vi "ME_acquire_21_HallSensor.vi"() -> ()   [LabVIEW 2015]
doc: "Use this template to build a producer/consumer design pattern. Use this template when you need to execute a process, such as data analysis, when a data source, such as a triggered acquisition, produces data at an uneven rate and you need to execute the process when the data becomes available."
uses:
  Mode.ctl
  oxford_driver/Oxford Drivers/BUSGEN.LLB/OxfordAddress.ctl
  <vilib>/Analysis/baseanly.llb/Mean (DBL).vi
  <vilib>/DAQmx/read.llb/DAQmx Read (Analog 1D DBL 1Chan NSamp).vi
  <vilib>/DAQmx/create/channels.llb/DAQmx Create Channel (AI-Voltage-Basic).vi
  <vilib>/DAQmx/configure/timing.llb/DAQmx Timing (Sample Clock).vi
  <vilib>/Utility/file.llb/Write Delimited Spreadsheet (DBL).vi
  <vilib>/DAQmx/miscellaneous.llb/DAQmx Fill In Error Info.vi
  <vilib>/express/express arith-compare/Formula/XNode/ExpressFormulaBlockNode.xnode
  <vilib>/Analysis/NI_AALBase.lvlib
panel:
  out "B lag":cluster{dbl[], dbl[]}(graph)
  out "T array":dbl[](array[numeric])
  out "Averaged I(T)":dbl[][](array[numeric])
  in  "Averaged P(T)":dbl[][](array[numeric])
  out "remaining elements 2":T1(array[cluster])
  out "Actual mean":dbl format="%0.6f"
  in  "Averaged dt":dbl[][](array[numeric])
  in  "Averaged P(B)":dbl[][](array[numeric])
  out "LockInR":dbl
  out "deltaUaux":dbl
  out "Hall Resistance (Ohm)":dbl caption="Actual AuxV" step=0.1
  in  "Stop":bool
  out "SaveSweep":bool=TRUE
  out "Measurement File_dn":path
  out "Measurement File_up":path
  out "Measurement File_average":path
  out "Actual Polarization":dbl
  in  "Reset IB?":bool
  in  "First?":bool
  in  "Save Period":dbl=1.0
  out "Averaged I(B)":dbl[][](array[numeric])
  out "P(uC/mm^2)":dbl[](array[numeric])
  in  "Sweep":bool
  out "Offset array":dbl[](array[numeric])
  in  "stop 2":bool
  in  "dB":dbl=0.005
  out "Actual B Field (T)":dbl
  out "Actual Temperature (K)":dbl
  out "Actual Current (pA)":dbl
  in  "Tab Control":T2(tab)
  in  "dt (K)":dbl=0.1
  in  "Max temperature (K)":dbl=20.0
  in  "Min Temperature (K)":dbl=4.5
  out "P(T)":cluster{"yi":dbl[], dbl[]}(graph)
  out "I(T)":cluster{dbl[], dbl[]}(graph)
  in  "Set temperature (K)":dbl=4.5
  in  "Temp Ramping Rate (K/min)":dbl=10.0
  in  "Heater Range":enum16{"Off", "Low", "Medium", "High"}(ring)
  in  "Heater On/Off":bool
  out "Setpoint Temperature (K)":dbl
  out "I(T) /Averaged/":cluster{"B array":dbl[], dbl[]}[](graph)
  out "P(T) /Averaged/":cluster{"B array":dbl[], dbl[]}[](graph)
  out "Up/Down 2":bool
  out "I(B) 3":cluster{dbl[], dbl[]}[](graph)
  out "I(B) /Averaged/":cluster{"B array":dbl[], dbl[]}[](graph)
  out "P(B) /Averaged/":cluster{"B array":dbl[], dbl[]}[](graph)
  out "P(B)":cluster{"yi":dbl[], dbl[]}(graph)
  in  "Set Field (T)":dbl
  in  "Go to Set":bool
  in  "Sweep Rate (T/min)":dbl=2.0 format="%.6f"
  in  "Field To Zero":bool
  out "Target Field":dbl
  in  "Min Field (T)":dbl
  in  "Max Field (T)":dbl=0.15
  in  "Threshold B (T)":dbl
  out "Up/Down":bool
  in  "Magnetic Field array (T)":dbl[](array[numeric])=[0.025, 0.05, 0.075, 0.1, 0.125, 0.15, 0.175, 0.2, 0.225, 0.25, 0.275, 0.3]
  in  "T Sweep Rate Array":dbl[](array[numeric])=[10.0, 20.0]
  in  "Max count array":i32[](array[numeric])=[2, 1, 0, 0, 0, 9, 10, 11, 12]
  in  "secs to wait":dbl=180.0
  out "Wait (s)":dbl
  in  "Directory":string
  out "Finished":bool=TRUE
  out "Step Rate":bool
  out "New":bool=TRUE
  in  "Temperature Array":dbl[](array[numeric])=[4.5, 5.0, 6.0, 7.0, 8.0, 9.0, 10.0, 11.0, 12.0]
  in  "Sweep Rate Array":dbl[](array[numeric])=[2.0, 1.0, 0.5, 0.1, 0.05, 9.0, 10.0, 11.0, 12.0]
  in  "Record ALL":bool
  in  "Max Countl":i32
  out "i":i32
  out "j":i32
  out "Step Temp":bool
  in  "FileName":string
  in  "Measure Noise":bool
  in  "Cycles":i32
  in  "maximum value":dbl=10.0 format="%0.2f"
  in  "minimum value":dbl=-10.0 format="%0.2f"
  in  "physical channels":tag="Dev1/ai1"
  out "PSD (pA/Hz^1/2) Peaks Removed":cluster{"f0":dbl, "df":dbl, "magnitude":dbl[]}(graph)
  out "PSD (pA/Hz^1/2)":cluster{"f0":dbl, "df":dbl, "magnitude":dbl[]}(graph)
  out "Current (pA) Filtered":waveform(dbl)(graph)
  out "Current (pA)":dbl[](graph)
  in  "Samples per channel":i32=1000
  in  "Rate":dbl=1000.0 format="%0.2f"
  in  "Cut-Off Frequency":dbl=100.0 caption="Lower Cut-Off"
  in  "Filter On":bool
  in  "Keithley (IV conv) averaging":i32=10
  in  "Lock_in_Amplifier":refnum<visa-resource-name>="GPIB0::5::INSTR"
  out "Dc offset":dbl
  in  "Calibrate":bool
  in  "IV converter":refnum<visa-resource-name>="GPIB0::20::INSTR"
  in  "Magnetic Field":refnum<visa-resource-name>="GPIB0::19::INSTR"
  out "Time Lag":dbl=0.0500025749206543
  in  "Lake Shore":refnum<visa-resource-name>="GPIB0::11::INSTR"
  in  "Temp Refresh (s)":dbl=0.1
  in  "Sampling rate (Hz)":dbl=10.0
  in  "Gain (V/A)":dbl=1000000000.0
  in  "Sample area (mm^2)":dbl=1.0
  out "Calibration Curve":cluster{dbl[], "Best Linear Fit":dbl[]}[](graph)=[{[0.0, 0.005, 0.01, 0.015, 0.02, 0.025, 0.03, 0.035, 0.04, 0.045, 0.05, 0.055, 0.06, 0.065, 0.07, 0.075, 0.08, 0.085, 0.09, 0.095, 0.1, 0.105, 0.11, 0.115, 0.12, 0.125, 0.13, 0.135, 0.14, 0.145, 0.15, 0.155, 0.16, 0.165, 0.17, 0.175, 0.18, 0.185, 0.19, 0.195, 0.2, 0.205, 0.21, 0.215, 0.22, 0.225, 0.23, 0.235, 0.24, 0.245, 0.25, 0.255, 0.26, 0.265, 0.27, 0.275, 0.28, 0.285, 0.29, 0.295, 0.3, 0.305, 0.31, 0.315, 0.32, 0.325, 0.33, 0.335, 0.34, 0.345, 0.35, 0.355, 0.36, 0.365, 0.37, 0.375, 0.38, 0.385, 0.39, 0.395, 0.4, 0.405, 0.41, 0.415, 0.42, 0.425, 0.43, 0.435, 0.44, 0.445, 0.45, 0.455, 0.46, 0.465, 0.47, 0.475, 0.48, 0.485, 0.49, 0.495, 0.5], "Best Linear Fit"=[-1.7e-06, 1.18e-05, 3.66e-05, 6.17e-05, 9.39e-05, 0.000122, 0.0001511, 0.0001781, 0.0002061, 0.0002355, 0.0002616, 0.0002895, 0.0003184, 0.0003446, 0.0003689, 0.0003958, 0.0004207, 0.0004464, 0.0004684, 0.0004953, 0.0005218, 0.0005459, 0.0005692, 0.0005897, 0.0006131, 0.0006347, 0.0006589, 0.0006834, 0.0007035, 0.0007249, 0.0007465, 0.000765, 0.0007858, 0.0008103, 0.0008302, 0.0008467, 0.000868, 0.0008855, 0.0009079, 0.0009248, 0.0009452, 0.0009633, 0.0009828, 0.0009992, 0.0010189, 0.0010338, 0.001054, 0.0010692, 0.0010858, 0.0011036, 0.0011162, 0.0011356, 0.0011502, 0.0011643, 0.0011834, 0.0011985, 0.0012131, 0.0012277, 0.0012423, 0.0012571, 0.0012691, 0.0012827, 0.0012976, 0.001313, 0.0013264, 0.0013388, 0.0013518, 0.0013638, 0.0013782, 0.0013909, 0.0014035, 0.0014175, 0.0014295, 0.0014407, 0.0014538, 0.0014641, 0.0014752, 0.0014861, 0.0014978, 0.0015081, 0.0015203, 0.001532, 0.0015422, 0.0015526, 0.001563, 0.0015754, 0.0015844, 0.0015955, 0.0016056, 0.001614, 0.0016239, 0.0016342, 0.0016457, 0.0016542, 0.0016635, 0.001674, 0.001681, 0.0016886, 0.0016986, 0.0017063, 0.0017155]}, {[0.0, 0.005, 0.01, 0.015, 0.02, 0.025, 0.03, 0.035, 0.04, 0.045, 0.05, 0.055, 0.06, 0.065, 0.07, 0.075, 0.08, 0.085, 0.09, 0.095, 0.1, 0.105, 0.11, 0.115, 0.12, 0.125, 0.13, 0.135, 0.14, 0.145, 0.15, 0.155, 0.16, 0.165, 0.17, 0.175, 0.18, 0.185, 0.19, 0.195, 0.2, 0.205, 0.21, 0.215, 0.22, 0.225, 0.23, 0.235, 0.24, 0.245, 0.25, 0.255, 0.26, 0.265, 0.27, 0.275, 0.28, 0.285, 0.29, 0.295, 0.3, 0.305, 0.31, 0.315, 0.32, 0.325, 0.33, 0.335, 0.34, 0.345, 0.35, 0.355, 0.36, 0.365, 0.37, 0.375, 0.38, 0.385, 0.39, 0.395, 0.4, 0.405, 0.41, 0.415, 0.42, 0.425, 0.43, 0.435, 0.44, 0.445, 0.45, 0.455, 0.46, 0.465, 0.47, 0.475, 0.48, 0.485, 0.49, 0.495, 0.5], "Best Linear Fit"=[-1.7e-06, 1.18e-05, 3.66e-05, 6.17e-05, 9.39e-05, 0.000122, 0.0001511, 0.0001781, 0.0002061, 0.0002355, 0.0002616, 0.0002895, 0.0003184, 0.0003446, 0.0003689, 0.0003958, 0.0004207, 0.0004464, 0.0004684, 0.0004953, 0.0005218, 0.0005459, 0.0005692, 0.0005897, 0.0006131, 0.0006347, 0.0006589, 0.0006834, 0.0007035, 0.0007249, 0.0007465, 0.000765, 0.0007858, 0.0008103, 0.0008302, 0.0008467, 0.000868, 0.0008855, 0.0009079, 0.0009248, 0.0009452, 0.0009633, 0.0009828, 0.0009992, 0.0010189, 0.0010338, 0.001054, 0.0010692, 0.0010858, 0.0011036, 0.0011162, 0.0011356, 0.0011502, 0.0011643, 0.0011834, 0.0011985, 0.0012131, 0.0012277, 0.0012423, 0.0012571, 0.0012691, 0.0012827, 0.0012976, 0.001313, 0.0013264, 0.0013388, 0.0013518, 0.0013638, 0.0013782, 0.0013909, 0.0014035, 0.0014175, 0.0014295, 0.0014407, 0.0014538, 0.0014641, 0.0014752, 0.0014861, 0.0014978, 0.0015081, 0.0015203, 0.001532, 0.0015422, 0.0015526, 0.001563, 0.0015754, 0.0015844, 0.0015955, 0.0016056, 0.001614, 0.0016239, 0.0016342, 0.0016457, 0.0016542, 0.0016635, 0.001674, 0.001681, 0.0016886, 0.0016986, 0.0017063, 0.0017155]}]
  in  "Offset?":bool
  in  "Magnet":bool=TRUE
  in  "Ramp":bool=TRUE
  in  "DaQ":bool
  in  "Moving average":i8=10
  in  "Sample Rate":dbl=1000.0
  in  "Number of Samples":i32=100
  in  "Physical Channel":tag="kartya/ai0"
  in  "Min Voltage":dbl=-5.0
  in  "Max Voltage":dbl=5.0
  in  "Terminal Configuration":i32(ring)=-1 items=["default"=-1, "RSE"=10083, "NRSE"=10078, "Differential"=10106, "Pseudodifferential"=12529]
  out "Confirm":bool
  in  "Dwell Time (ms)":u32=1000
  out "Calibration Curve Data":dbl[][](array[numeric])=[[0.0, 0.005, 0.01, 0.015, 0.02, 0.025, 0.03, 0.035, 0.04, 0.045, 0.05, 0.055, 0.06, 0.065, 0.07, 0.075, 0.08, 0.085, 0.09, 0.095, 0.1, 0.105, 0.11, 0.115, 0.12, 0.125, 0.13, 0.135, 0.14, 0.145, 0.15, 0.155, 0.16, 0.165, 0.17, 0.175, 0.18, 0.185, 0.19, 0.195, 0.2, 0.205, 0.21, 0.215, 0.22, 0.225, 0.23, 0.235, 0.24, 0.245, 0.25, 0.255, 0.26, 0.265, 0.27, 0.275, 0.28, 0.285, 0.29, 0.295, 0.3, 0.305, 0.31, 0.315, 0.32, 0.325, 0.33, 0.335, 0.34, 0.345, 0.35, 0.355, 0.36, 0.365, 0.37, 0.375, 0.38, 0.385, 0.39, 0.395, 0.4, 0.405, 0.41, 0.415, 0.42, 0.425, 0.43, 0.435, 0.44, 0.445, 0.45, 0.455, 0.46, 0.465, 0.47, 0.475, 0.48, 0.485, 0.49, 0.495, 0.5], [-1.7e-06, 1.18e-05, 3.66e-05, 6.17e-05, 9.39e-05, 0.000122, 0.0001511, 0.0001781, 0.0002061, 0.0002355, 0.0002616, 0.0002895, 0.0003184, 0.0003446, 0.0003689, 0.0003958, 0.0004207, 0.0004464, 0.0004684, 0.0004953, 0.0005218, 0.0005459, 0.0005692, 0.0005897, 0.0006131, 0.0006347, 0.0006589, 0.0006834, 0.0007035, 0.0007249, 0.0007465, 0.000765, 0.0007858, 0.0008103, 0.0008302, 0.0008467, 0.000868, 0.0008855, 0.0009079, 0.0009248, 0.0009452, 0.0009633, 0.0009828, 0.0009992, 0.0010189, 0.0010338, 0.001054, 0.0010692, 0.0010858, 0.0011036, 0.0011162, 0.0011356, 0.0011502, 0.0011643, 0.0011834, 0.0011985, 0.0012131, 0.0012277, 0.0012423, 0.0012571, 0.0012691, 0.0012827, 0.0012976, 0.001313, 0.0013264, 0.0013388, 0.0013518, 0.0013638, 0.0013782, 0.0013909, 0.0014035, 0.0014175, 0.0014295, 0.0014407, 0.0014538, 0.0014641, 0.0014752, 0.0014861, 0.0014978, 0.0015081, 0.0015203, 0.001532, 0.0015422, 0.0015526, 0.001563, 0.0015754, 0.0015844, 0.0015955, 0.0016056, 0.001614, 0.0016239, 0.0016342, 0.0016457, 0.0016542, 0.0016635, 0.001674, 0.001681, 0.0016886, 0.0016986, 0.0017063, 0.0017155]]
  in  "Temp/Magnetic Field":bool
  out "index":i8
  out "Read?":bool
  out "Magnetic Field (T)":dbl[](array[numeric])
  out "Reset":bool
  out "Measured Current (pA)":dbl[](array[numeric])
  out "Elapsed Time (s)":dbl[](array[numeric])
  out "Start time":timestamp
  in  "Enum":T3=enum."Process"
  out "B array":dbl[](array[numeric])
  in  "dB (T)":dbl=0.0025
  in  "Counter":i8
  out "L magnet (H)":dbl
  out "R magnet (mOhm)":dbl
  out "Actual Current (R0)":dbl
  out "Nominal Field (T)":dbl
  out "Temperature array":dbl[](array[numeric])
  in  "New Measurement File":bool
  out "Measurement File":path
  out "refnum out":refnum<file>
  in  "Measuring":bool
  in  "Measure /Pause":bool
  in  "stop":bool
  # "DeltaForce"
  # "Discrete"
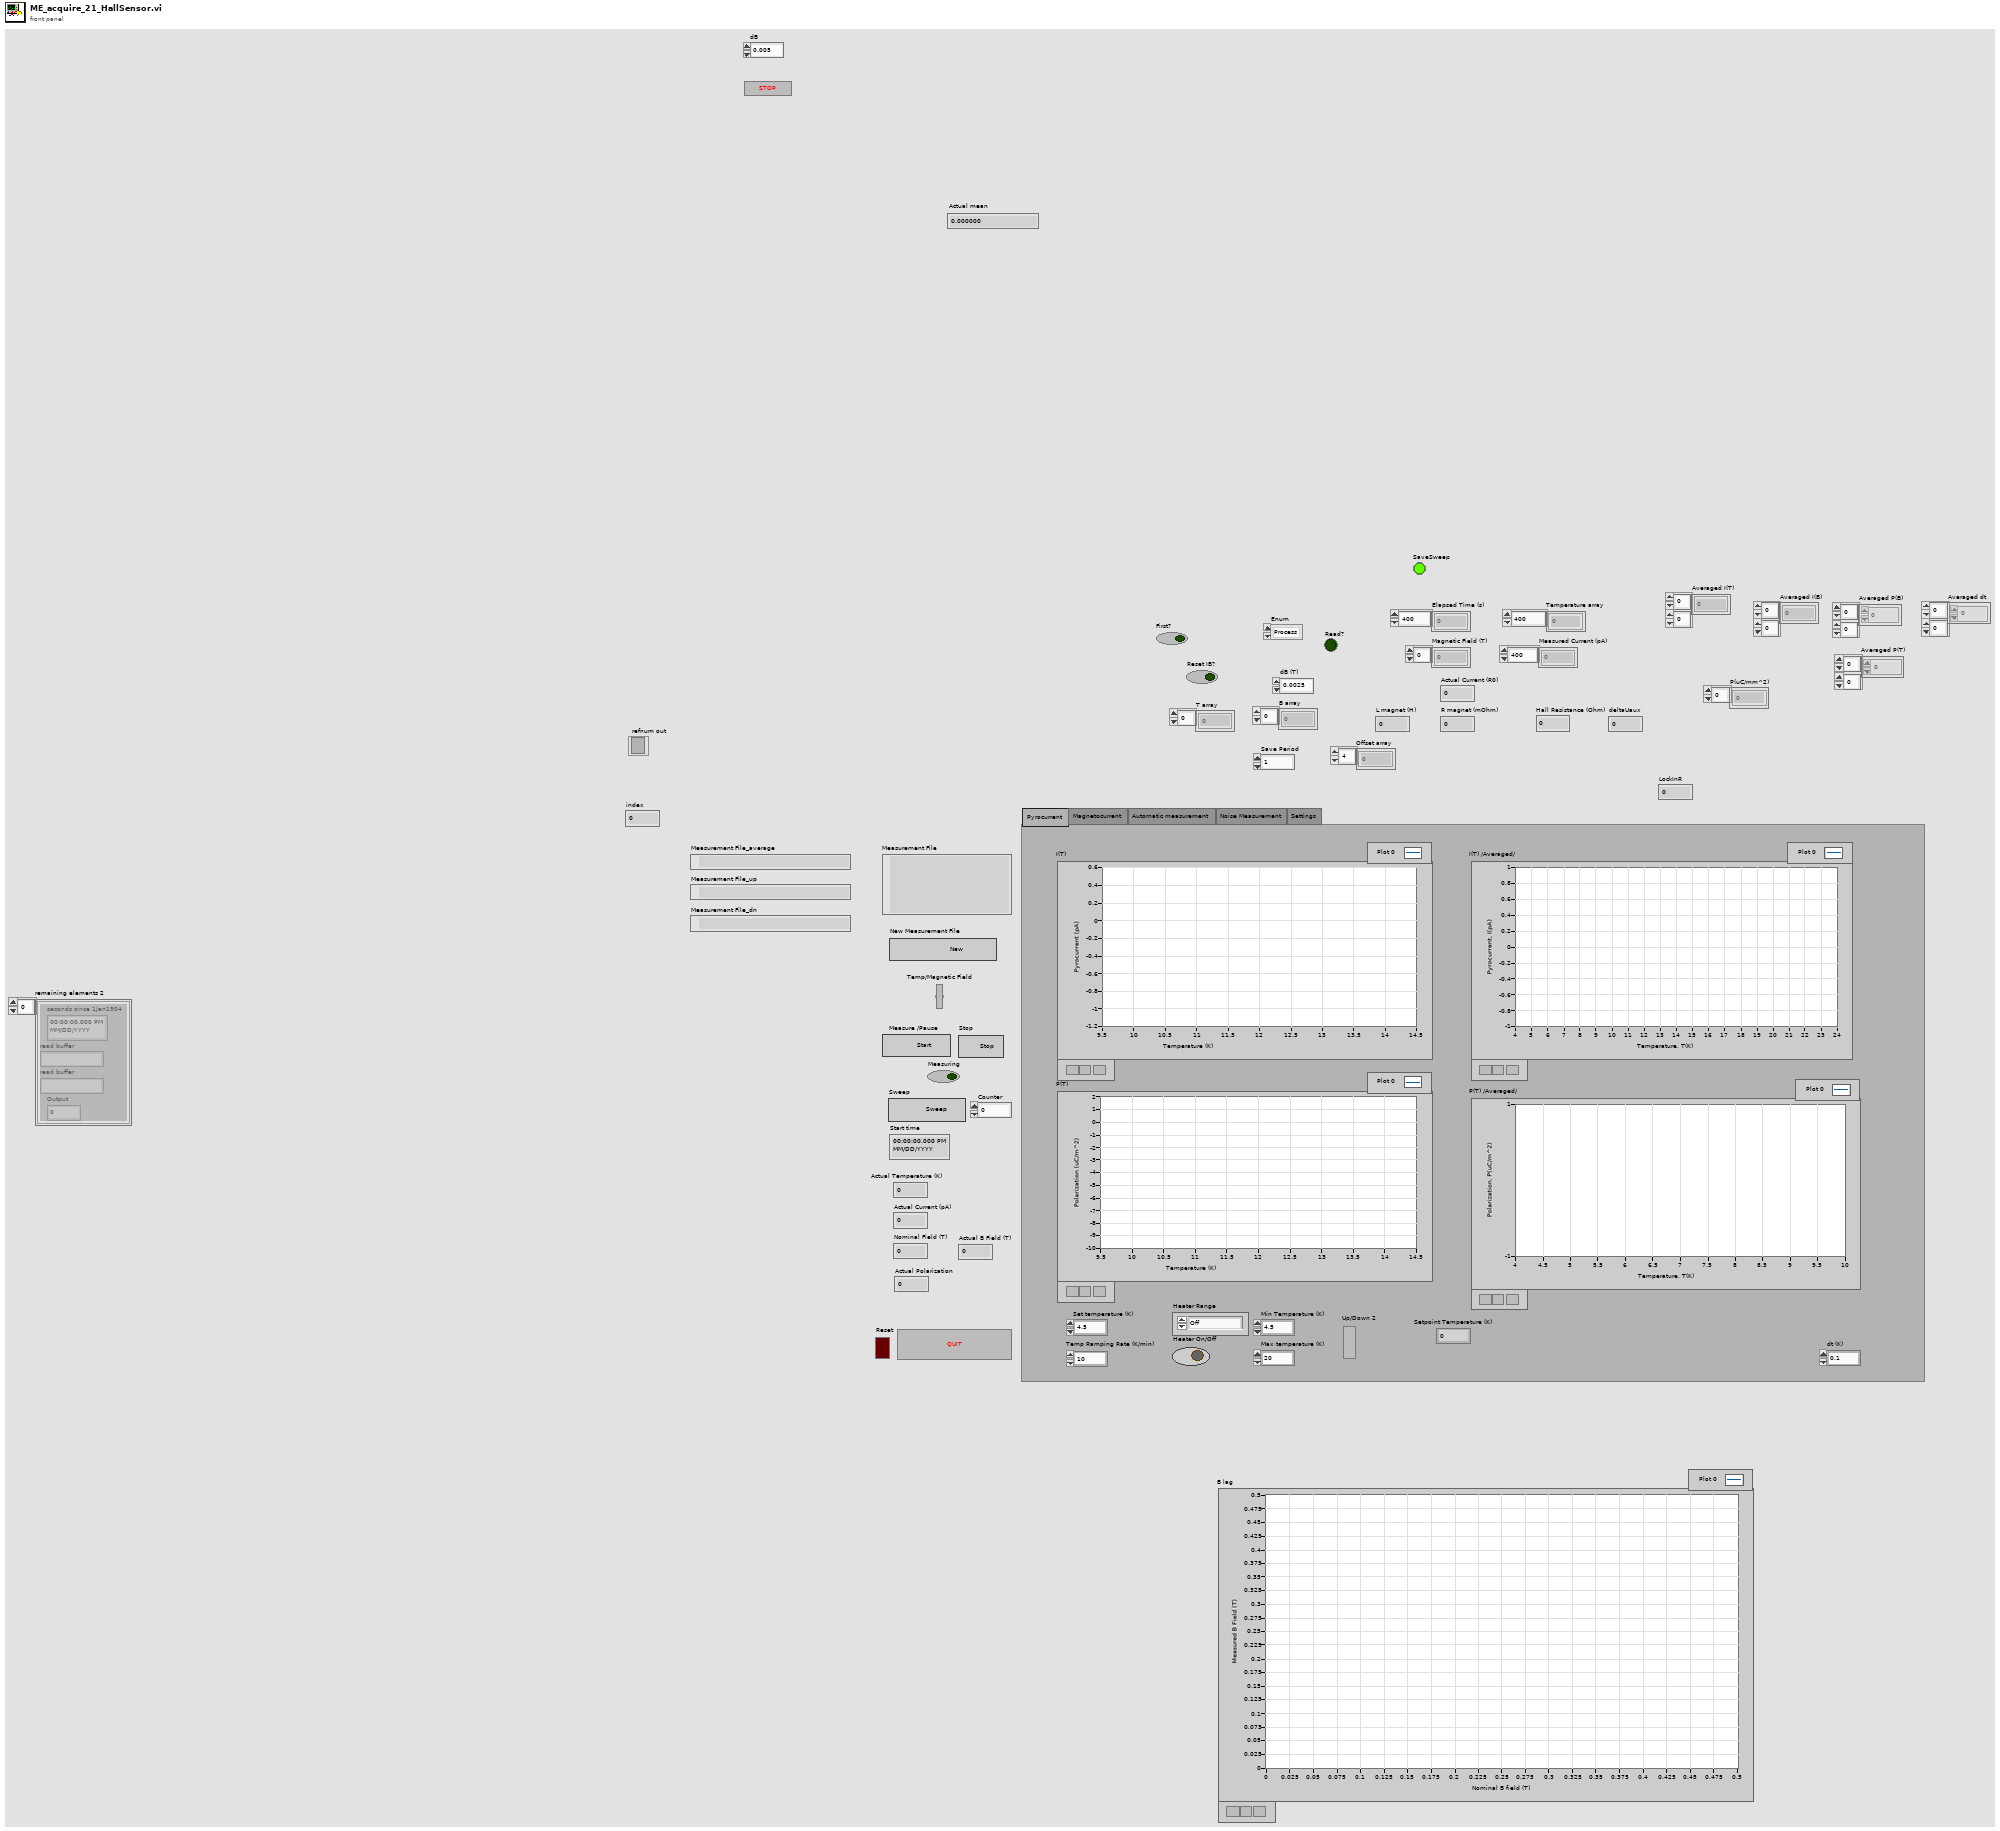
[diagram p1: front panel]
types:
  T1 = cluster{"seconds since 1Jan1904":timestamp, "read buffer":string, "read buffer":string, "Output":dbl}[]
  T2 = enum32{"Pyrocurrent", "Magnetocurrent", "Automatic measurement", "Noise Measurement", "Settings"}
  T3 = typedef "Mode.ctl" = enum16{"Offset", "Process", "Sweep", "StepOxford", "StepDelta", "Plot", "Save", "New", "Return", ""}
  T4 = cluster{"seconds since 1Jan1904":timestamp, "read buffer":string, "read buffer":string, "Output":dbl}
  T5 = enum16{"open", "replace", "create", "open or create", "replace or create", "replace or create with confirmation"}
  T6 = typedef "OxfordAddress.ctl" = cluster{"Com Port":i32, "ISOBUS Address":i32, "GPIB Address":i16, "Communication":enum16{"RS232", "ISOBUS", "GPIB", "Gateway"}}
  T7 = cluster{"B array":dbl[], "Averaged P(B) Out":dbl[]}
  T8 = cluster{"B array":dbl[], "BaselineSubtracted I(B)":dbl[]}
  T9 = cluster{"B array":dbl[], "Averaged P(B) Out":dbl[]}[]
  T10 = cluster{"B array":dbl[], "BaselineSubtracted I(B)":dbl[]}[]
  T11 = cluster{"T array":dbl[], "Averaged P(T) Out":dbl[]}
  T12 = cluster{"T array":dbl[], "Averaged I(B) out":dbl[]}
  T13 = cluster{"T array":dbl[], "Averaged P(T) Out":dbl[]}[]
  T14 = cluster{"T array":dbl[], "Averaged I(B) out":dbl[]}[]
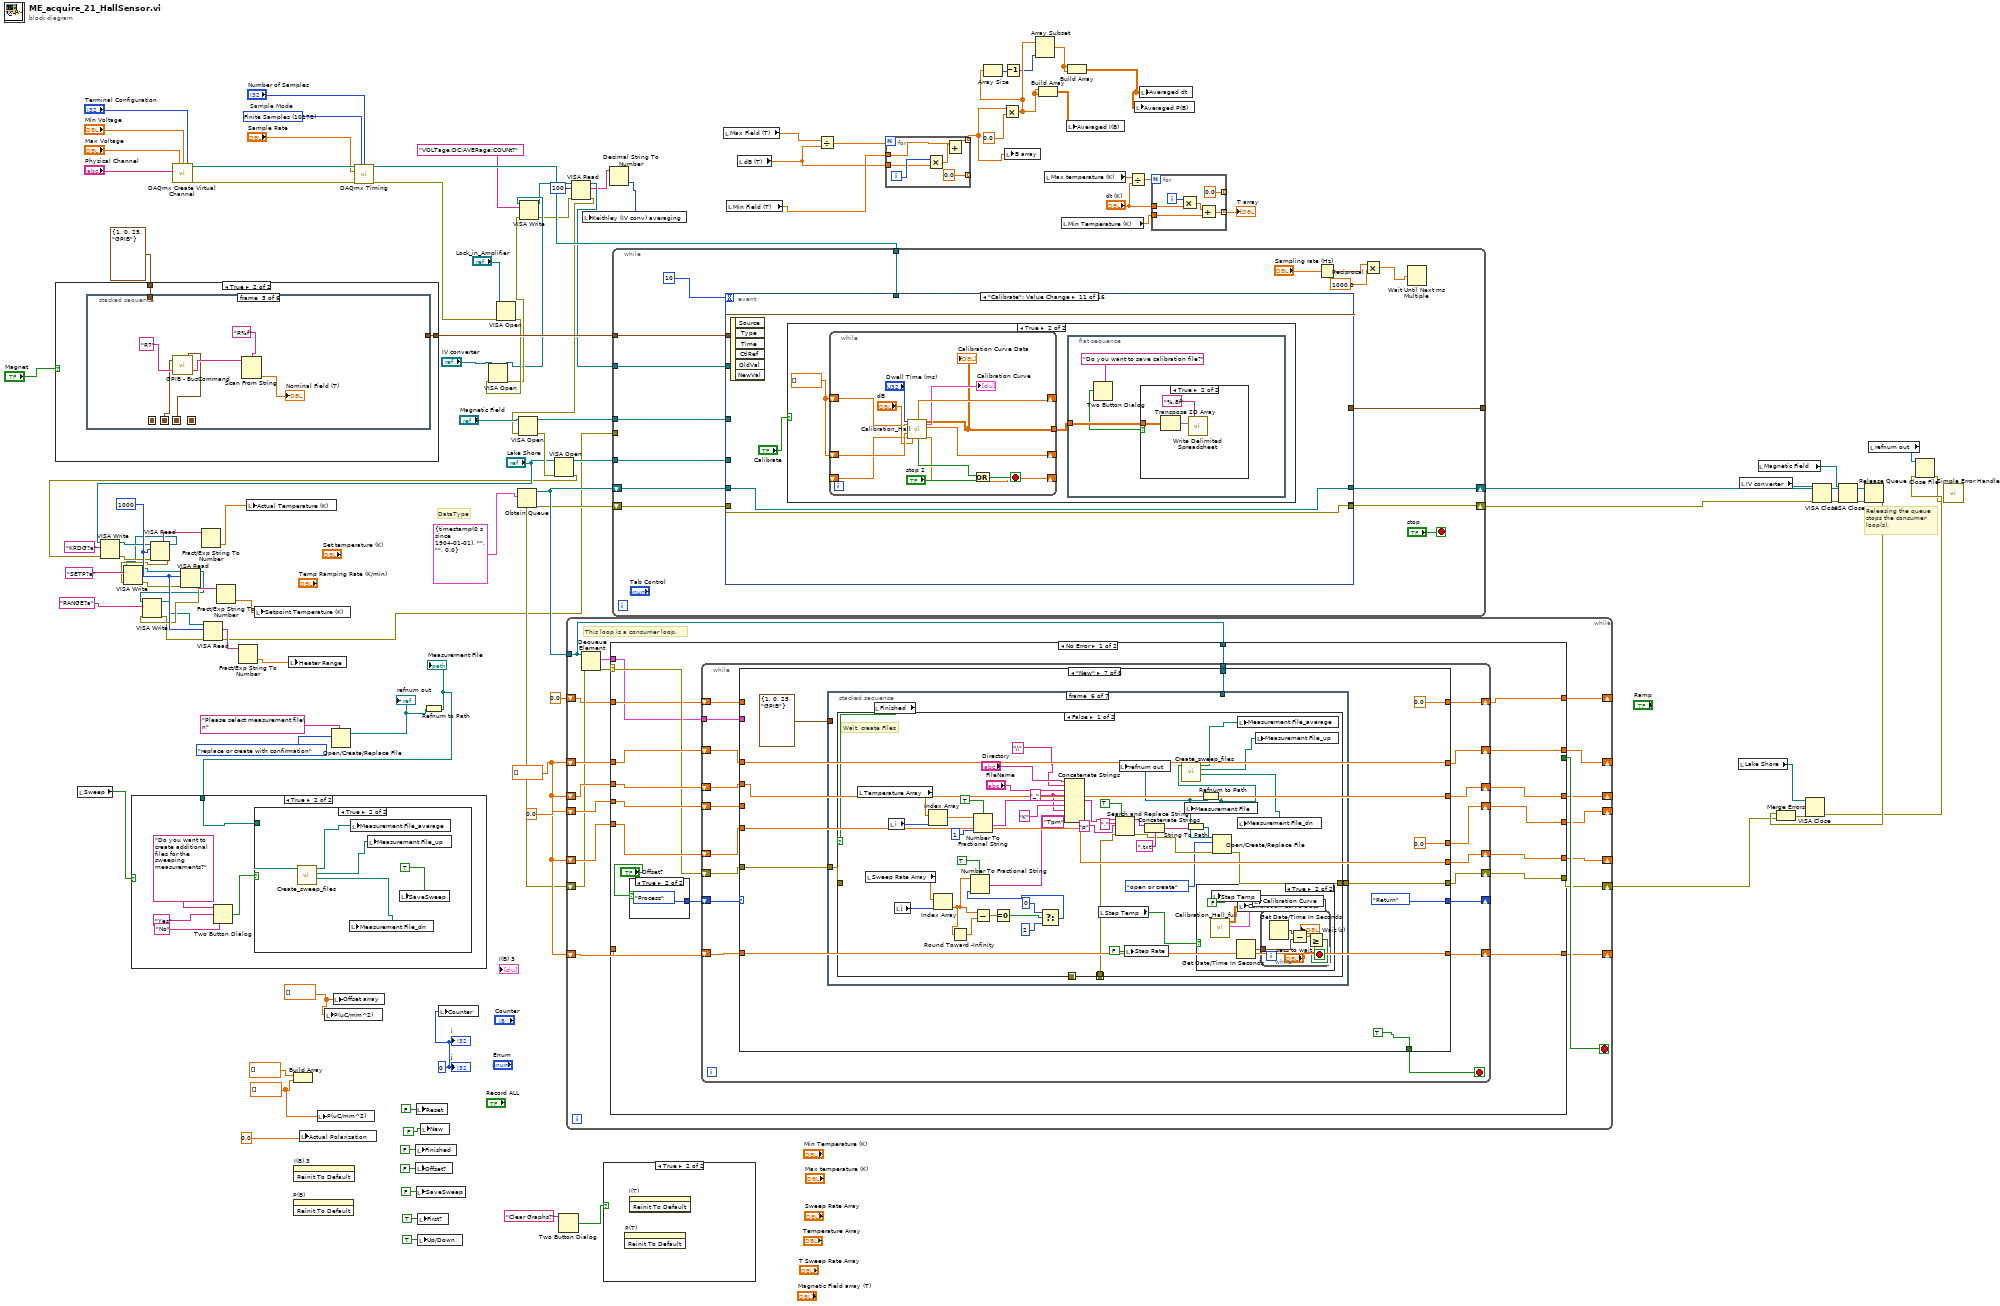
[diagram p0: block diagram]
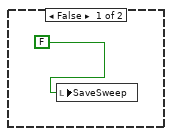
[diagram p4: hidden frame]
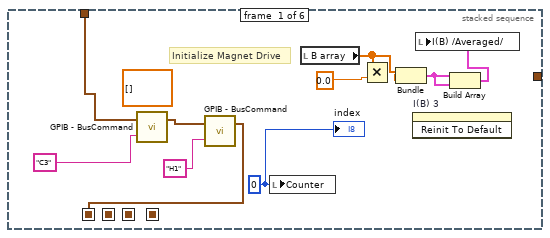
[diagram p6: hidden frame]
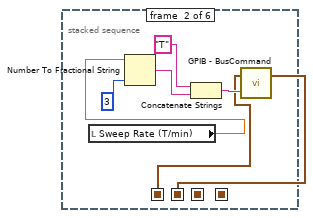
[diagram p7: hidden frame]
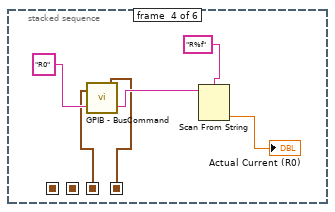
[diagram p8: hidden frame]
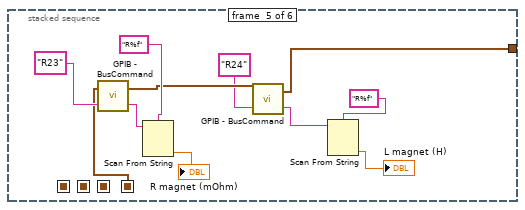
[diagram p9: hidden frame]
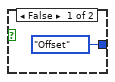
[diagram p11: hidden frame]
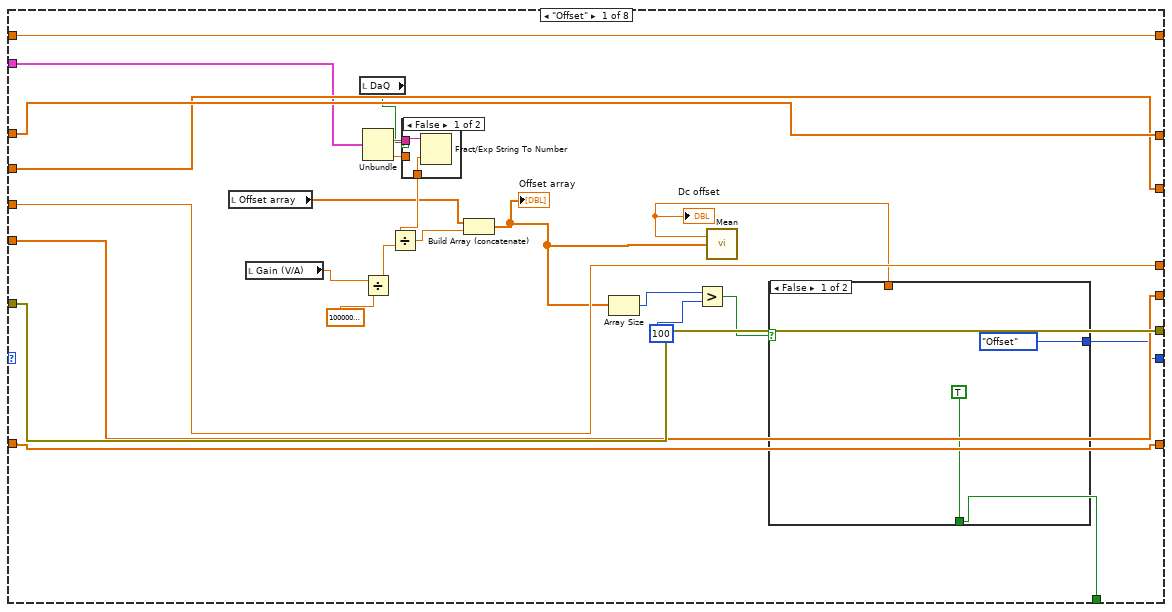
[diagram p12: hidden frame]
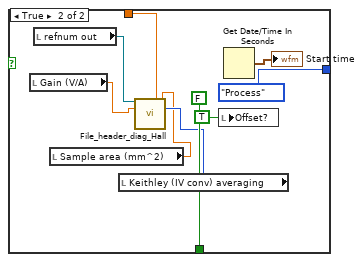
[diagram p14: hidden frame]
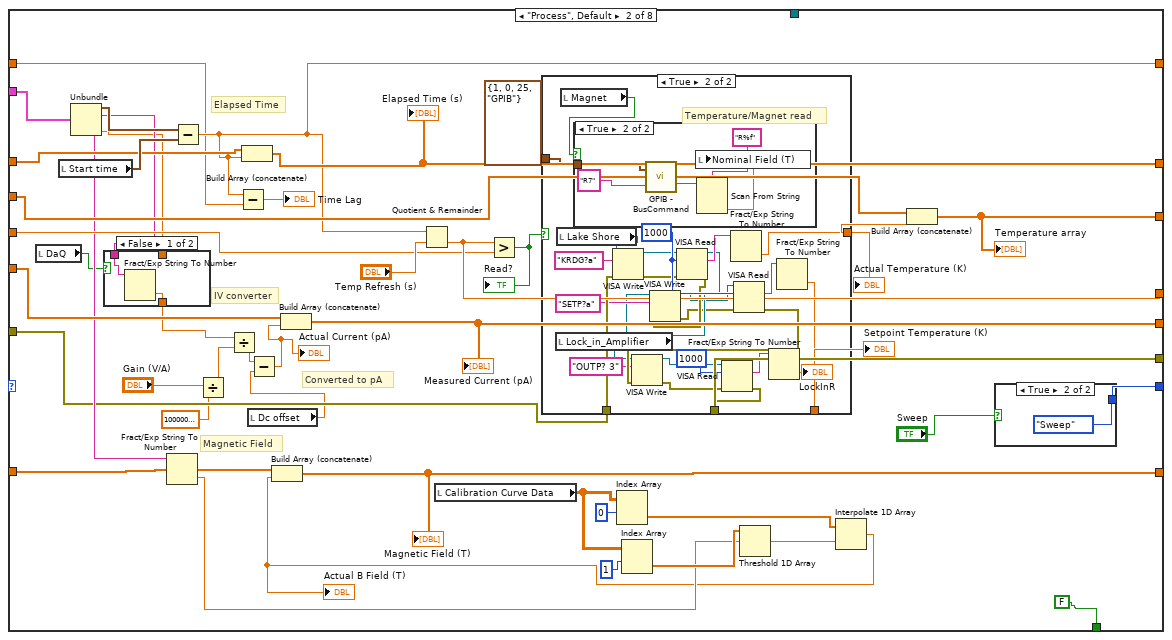
[diagram p15: hidden frame]
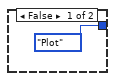
[diagram p17: hidden frame]
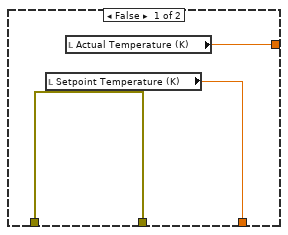
[diagram p18: hidden frame]
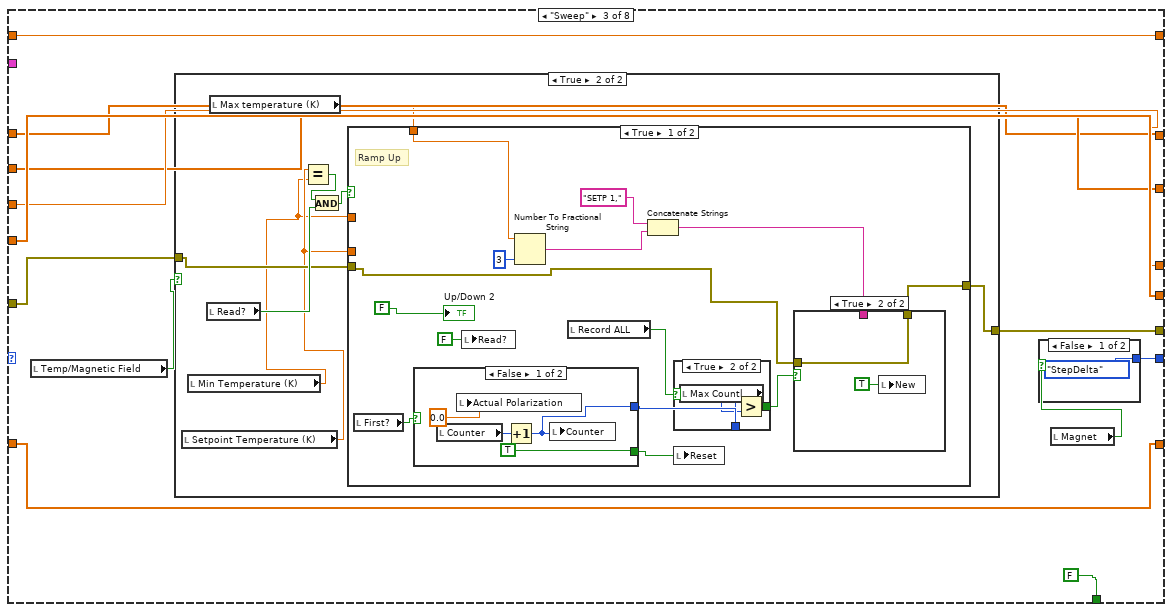
[diagram p20: hidden frame]
diagram:
  w27 = 10178 items=["Finite Samples"=10178, "Continuous Samples"=10123, "Hardware Timed Single Point"=12522]  # Sample Mode
  w54 = u32 1000 ("byte count")
  w65 = 0 ("j")
  w62 = dbl[] []
  w80 = dbl[] []
  w86 = dbl[] []
  # "DataType"
  # "Releasing the queue stops the consumer loop(s)."
  n1 = case shown="True" "Magnet" {
    tunnel: T6 {"Com Port"=1, "ISOBUS Address"=0, "GPIB Address"=25, "Communication"=enum."GPIB"} ("Address") -> [w110 w112]
    tunnel: [w110 w111] -> w92
    frame False {
    }
    frame True {
      n2 = stacked-sequence {
        seq-local: [w120 _ _ _ _ _] -> [_ w125 _ _ _ _]
        seq-local: [_ w124 _ _ _ _] -> [_ _ w132 _ _ _]
        seq-local: [_ _ w131 _ _ _] -> [_ _ _ w138 _ _]
        seq-local: [_ _ _ w137 _ _] -> [_ _ _ _ w149 _]
        tunnel: w112 -> [w122 _ _ _ _ _]
        tunnel: [_ _ _ _ w147 _] -> w111
        frame #0 {
          (unwired) dbl[][] []
          w118 = i8 0 ("Counter")
          # "Initialize Magnet Drive"
          n3 = call "GPIB - BusCommand.vi"("Command"="C3", "Address"=w122) -> ("Address(thru)"=w121:T6)  [unwired: 1 out]
          n4 = call "GPIB - BusCommand.vi"("Command"="H1", "Address"=w121) -> ("Address(thru)"=w120:T6)  [unwired: 1 out]
          n5 = local write "Counter"(w118) -> ()
          n6 = local read "B array"() -> (w116:dbl[])
          n7 = Multiply(x=w116, y=0.0) -> (x*y=w115:dbl[])
          n8 = Bundle("B array"=w116, w115) -> (w114:cluster{"B array":dbl[], dbl[]})  [unwired: 1 in]
          n9 = invoke on="I(B) 3" class="XYGraph (strict)" method="Reinit To Default"() -> ()  [unwired: 3 in, 3 out]
          n10 = Build Array(w114, w114) -> (w113:cluster{"B array":dbl[], dbl[]}[])
          n11 = local write "I(B) /Averaged/"(w113) -> ()
          "index" <- w118
        }
        frame #1 {
          n12 = local read "Sweep Rate (T/min)"() -> (w126:dbl)
          n13 = Number To Fractional String(number=w126, precision (6)=i16 3) -> (F-format string=w128:string)  [unwired: 2 in]
          n14 = Concatenate Strings("T" ("format string"), w128) -> (w127:string)
          n15 = call "GPIB - BusCommand.vi"("Command"=w127, "Address"=w125) -> ("Address(thru)"=w124:T6)  [unwired: 1 out]
        }
        frame #2 {
          n16 = call "GPIB - BusCommand.vi"("Command"="R7" ("format string"), "Address"=w132) -> ("Reply"=w136:string, "Address(thru)"=w131:T6)
          n17 = Scan From String(format string="R%f" ("remaining string"), input string=w136) -> (output 1=→"Nominal Field (T)":dbl)  [unwired: 3 in, 3 out]
        }
        frame #3 {
          n18 = call "GPIB - BusCommand.vi"("Command"="R0" ("format string"), "Address"=w138) -> ("Reply"=w142:string, "Address(thru)"=w137:T6)
          n19 = Scan From String(format string="R%f" ("remaining string"), input string=w142) -> (output 1=→"Actual Current (R0)":dbl)  [unwired: 3 in, 3 out]
        }
        frame #4 {
          n20 = call "GPIB - BusCommand.vi"("Command"="R23" ("format string"), "Address"=w149) -> ("Reply"=w153:string, "Address(thru)"=w148:T6)
          n21 = Scan From String(format string="R%f" ("remaining string"), input string=w153) -> (output 1=→"R magnet (mOhm)":dbl)  [unwired: 3 in, 3 out]
          n22 = call "GPIB - BusCommand.vi"("Command"="R24" ("format string"), "Address"=w148) -> ("Reply"=w145:string, "Address(thru)"=w147:T6)
          n23 = Scan From String(format string="R%f" ("remaining string"), input string=w145) -> (output 1=→"L magnet (H)":dbl)  [unwired: 3 in, 3 out]
        }
        frame #5 {
        }
      }
    }
  }
  n24 = local read "Sweep"() -> (w70:bool)
  n25 = call-poly <vilib>:"DAQmx Create Virtual Channel.vi"("maximum value"="Max Voltage", "minimum value"="Min Voltage", "input terminal configuration"="Terminal Configuration", "physical channels"="Physical Channel") -> ("task out"=w25:refnum<k21>, "error out"=w26:errorcluster)  [unwired: 10 in]
  n26 = Build Array(dbl[] [], w62) -> ()  [unwired: 1 out]
  n27 = invoke on="P(B)" class="XYGraph (strict)" method="Reinit To Default"() -> ()  [unwired: 3 in, 3 out]
  n28 = invoke on="I(B) 3" class="XYGraph (strict)" method="Reinit To Default"() -> ()  [unwired: 3 in, 3 out]
  n29 = local write "Actual Polarization"(0.0 ("Actual Polarization")) -> ()
  n30 = local write "P(uC/mm^2)"(w62) -> ()
  n31 = local write "P(uC/mm^2)"(w80) -> ()
  n32 = Open/Create/Replace File(prompt="Please select measurement file\n", operation (0:open)=T5."replace or create with confirmation") -> (refnum out=w89:refnum<file>)  [unwired: 4 in, 2 out]
  "refnum out" <- w89
  n33 = local write "Offset array"(w80) -> ()
  n34 = call-poly <vilib>:"DAQmx Timing.vi"("task/channels in"=w25, "sample mode"=w27, "samples per channel"="Number of Samples", "rate"="Sample Rate", "error in"=w26) -> ("task out"=w17:refnum<k21>, "error out"=w18:errorcluster)  [unwired: 9 in]
  n35 = local write "Finished"(FALSE ("Finished")) -> ()
  n36 = local write "Offset?"(FALSE ("Offset?")) -> ()
  n37 = local write "Reset"(FALSE ("Reset")) -> ()
  n38 = local write "SaveSweep"(FALSE ("SaveSweep")) -> ()
  n39 = local write "First?"(TRUE ("First?")) -> ()
  n40 = local write "Up/Down"(TRUE ("Up/Down")) -> ()
  n41 = local write "New"(FALSE ("New")) -> ()
  n42 = Refnum to Path(1:w89) -> (0:w69:path)
  "Measurement File" <- w69
  n43 = case shown="True" w70 {
    tunnel: w69 -> [_ w154]
    frame False {
    }
    frame True {
      n44 = Two Button Dialog(message="Do you want to create additional files for the sweeping measurements?" ("string"), 1:"No" ("F button name (\"Cancel\")"), 2:"Yes" ("T button name (\"OK\")")) -> (T button?=w156:bool)
      n45 = case shown="True" w156 {
        tunnel: w154 -> [_ w164]
        frame False {
          n46 = local write "SaveSweep"(FALSE ("SaveSweep")) -> ()
        }
        frame True {
          n47 = call "Create_sweep_files.vi"("Measurement File"=w164) -> ("Path 3"=w161:path, "Path 2"=w162:path, "Path"=w163:path)  [unwired: 8 in]
          n48 = local write "Measurement File_dn"(w161) -> ()
          n49 = local write "Measurement File_average"(w163) -> ()
          n50 = local write "Measurement File_up"(w162) -> ()
          n51 = local write "SaveSweep"(TRUE) -> ()
        }
      }
    }
  }
  n52 = local write "Counter"(w65) -> ()
  n53 = VISA Open(error in (no error)=w18, VISA resource name="Lock_in_Amplifier") -> (error out=w37:errorcluster)  [unwired: 3 in, 1 out]
  n54 = VISA Open(error in (no error)=w37, VISA resource name="IV converter") -> (VISA resource name=w14:refnum<visa-resource-name>, error out=w15:errorcluster)  [unwired: 3 in]
  n55 = Obtain Queue(element data type=T4 {"seconds since 1Jan1904"=timestamp(0 s since 1904-01-01), "read buffer"="", "read buffer"="", "Output"=0.0} ("output cluster")) -> (queue out=w109:refnum<queue>, error out=w84:errorcluster)  [unwired: 4 in, 1 out]
  n56 = VISA Write(VISA resource name=w14, write buffer="VOLTage:DC:AVERage:COUNt?", error in (no error)=w15) -> (VISA resource name out=w10:refnum<visa-resource-name>, error out=w12:errorcluster)  [unwired: 1 out]
  n57 = Two Button Dialog(message="Clear Graphs?") -> (T button?=w64:bool)  [unwired: 2 in]
  n58 = while {
    tunnel: w109 -> [w165]
    shift-right: [w178] -> _
    shift-left: w86 -> [w177]
    shift-right: [w176] -> _
    shift-left: w86 -> [w175]
    shift-right: [w174] -> _
    shift-left: w86 -> [w173]
    shift-right: [w172] -> _
    shift-left: 0.0 -> [w171]
    shift-right: [w170] -> _
    shift-left: w86 -> [w169]
    shift-right: [w179] -> w97
    shift-left: w84 -> [w168]
    shift-right: [w167] -> _
    shift-left: 0.0 -> [w166]
    stop <- w180 stop-if-true
    # "This loop is a consumer loop."
    n59 = Dequeue Element(queue=w165, error in (no error)=w168) -> (element=w181:T4, error out=w182:errorcluster)  [unwired: 1 in, 2 out]
    n60 = case shown="No Error" w182 {
      selector: w182 -> [w189 w898]
      tunnel: w181 -> [w183 _]
      tunnel: [_ TRUE] -> w180
      tunnel: [w188 w898] -> w179
      tunnel: [w199 w897] -> w178
      tunnel: w177 -> [w198 w897]
      tunnel: [w197 w894] -> w176
      tunnel: w175 -> [w196 w894]
      tunnel: [w195 w893] -> w174
      tunnel: w173 -> [w194 w893]
      tunnel: [w193 w895] -> w172
      tunnel: w171 -> [w192 w895]
      tunnel: [w191 w896] -> w170
      tunnel: w169 -> [w190 w896]
      tunnel: [w187 w892] -> w167
      tunnel: w166 -> [w186 w892]
      tunnel: w165 -> [w184 _]
      frame No Error {
        n61 = case shown="True" "Offset?" {
          tunnel: [Mode."Offset" ("Enum") Mode."Process" ("Enum")] -> w200
          frame False {
          }
          frame True {
          }
        }
        n62 = while {
          shift-right: [w209] -> _
          shift-left: w200 -> [w221]
          tunnel: w183 -> [w220]
          shift-right: [w219] -> w199
          shift-left: w198 -> [w218]
          shift-right: [w211] -> w191
          shift-left: w190 -> [w210]
          shift-right: [w213] -> w193
          shift-left: w192 -> [w212]
          shift-right: [w217] -> w197
          shift-left: w196 -> [w216]
          shift-right: [w207] -> w188
          shift-left: w189 -> [w208]
          shift-right: [w215] -> w195
          shift-left: w194 -> [w214]
          shift-right: [w205] -> w187
          shift-left: w186 -> [w204]
          tunnel: w184 -> [w203]
          stop <- w206 stop-if-true
          n63 = case shown="\"New\"" w221 {
            selector: w221 -> [_ _ _ _ _ _ _ w885]
            tunnel: w220 -> [w239 w302 _ _ _ _ _ _]
            tunnel: [w245 w299 w348 w482 w538 w611 w724 w890] -> w219
            tunnel: w218 -> [w245 w294 w348 w482 w538 w607 w724 w890]
            tunnel: [w240 w298 w351 w479 w540 w613 w722 w887] -> w217
            tunnel: w216 -> [w240 w297 w351 w479 w540 w608 w722 w887]
            tunnel: [w241 w296 w353 w477 w535 w614 w720 w884] -> w215
            tunnel: w214 -> [w241 w295 w353 w477 w535 w609 w720 w884]
            tunnel: [w243 w293 w350 w480 w536 w617 0.0 w888] -> w213
            tunnel: w212 -> [w243 w292 w350 w480 w536 w617 _ w888]
            tunnel: [w244 w289 w349 w481 w537 w612 w723 w889] -> w211
            tunnel: w210 -> [w244 w290 w349 w481 w537 w610 w723 w889]
            tunnel: [w228 w287 w346 Mode."Plot" ("Enum") Mode."Save" ("Enum") w618 Mode."Return" ("Enum") w885] -> w209
            tunnel: w208 -> [w242 w285 w355 w474 w543 w616 w716 w886]
            tunnel: [w242 w284 w354 w473 w543 w616 w715 w886] -> w207
            tunnel: [w224 FALSE FALSE FALSE FALSE w605 TRUE TRUE] -> w206
            tunnel: [w227 w281 w347 w475 w539 w615 0.0 w891] -> w205
            tunnel: w204 -> [w227 w280 w347 w475 w539 w615 _ w891]
            tunnel: w203 -> [_ _ _ _ _ _ w714 _]
            frame "Offset" {
              n64 = local read "Offset array"() -> (w233:dbl[])
              n65 = local read "Gain (V/A)"() -> (w237:dbl)
              n66 = local read "DaQ"() -> (w223:bool)
              n67 = Unbundle(w239) -> ("read buffer"=w226:string, "Output"=w222:dbl)  [unwired: 2 out]
              n68 = Divide(x=w237, y=1000000000000.0) -> (x/y=w235:dbl)
              n69 = case shown="False" w223 {
                tunnel: [w247 w248] -> w238
                tunnel: w226 -> [w246 _]
                tunnel: w222 -> [_ w248]
                frame False {
                  n70 = Fract/Exp String To Number(string=w246) -> (number=w247:dbl)  [unwired: 3 in, 1 out]
                }
                frame True {
                }
              }
              n71 = Divide(x=w238, y=w235) -> (x/y=w234:dbl)
              n72 = Build Array (concatenate)(w233, w234) -> (w229:dbl[])
              "Offset array" <- w229
              n73 = Array Size(array=w229) -> (size(s)=w232:i32)
              n74 = Greater?(x=w232, y=100) -> (0:w230:bool)
              n75 = call-poly <vilib>:"Mean.vi"("X"=w229) -> ("mean"=w225:dbl)  [unwired: 1 out]
              "Dc offset" <- w225
              n76 = case shown="False" w230 {
                tunnel: [Mode."Offset" ("Enum") Mode."Process" ("Enum")] -> w228
                tunnel: w225 -> [_ w255]
                tunnel: [TRUE FALSE] -> w224
                frame False {
                }
                frame True {
                  n77 = local read "Gain (V/A)"() -> (w256:dbl)
                  n78 = local read "refnum out"() -> (w257:refnum<file>)
                  n79 = local read "Sample area (mm^2)"() -> (w251:dbl)
                  n80 = local read "Keithley (IV conv) averaging"() -> (w252:i32)
                  n81 = call "File_header_diag_Hall.vi"("Byte Stream File in"=w257, "OFFSET"=w255, "Sample area"=w251, "Gain"=w256, "Averaging"=w252) -> ()  [unwired: 11 in]
                  n82 = local write "Offset?"(TRUE ("Offset?")) -> ()
                  n83 = Get Date/Time In Seconds() -> (seconds since 1Jan1904=→"Start time":timestamp)
                }
              }
            }
            frame "Process", Default {
              # "Converted to pA"
              # "Magnetic Field"
              # "IV converter"
              # "Elapsed Time"
              n84 = local read "DaQ"() -> (w270:bool)
              n85 = local read "Start time"() -> (w300:timestamp)
              n86 = Unbundle(w302) -> ("seconds since 1Jan1904"=w301:timestamp, "read buffer"=w271:string, "read buffer"=w286:string, "Output"=w268:dbl)
              n87 = case shown="False" w270 {
                tunnel: w271 -> [w306 _]
                tunnel: [w305 w307] -> w269
                tunnel: w268 -> [_ w307]
                frame False {
                  n88 = Fract/Exp String To Number(string=w306) -> (number=w305:dbl)  [unwired: 3 in, 1 out]
                }
                frame True {
                }
              }
              n89 = Fract/Exp String To Number(string=w286) -> (number=w263:dbl)  [unwired: 3 in, 1 out]
              n90 = Subtract(x=w301, y=w300) -> (x-y=w281:dbl)
              n91 = Divide(x="Gain (V/A)", y=1000000000000.0) -> (x/y=w279:dbl)
              n92 = Divide(x=w269, y=w279) -> (x/y=w276:dbl)
              n93 = Subtract(x=w281, y=w280) -> (x-y=→"Time Lag":dbl)
              n94 = Build Array (concatenate)(w294, w281) -> (w299:dbl[])
              "Elapsed Time (s)" <- w299
              n95 = local read "Dc offset"() -> (w274:dbl)
              n96 = Subtract(x=w276, y=w274) -> (x-y=w275:dbl)
              "Actual Current (pA)" <- w275
              n97 = Build Array (concatenate)(w297, w275) -> (w298:dbl[])
              "Measured Current (pA)" <- w298
              n98 = Quotient & Remainder(x=w281, y="Temp Refresh (s)") -> (floor(x/y)=w293:dbl)  [unwired: 1 out]
              n99 = local read "Calibration Curve Data"() -> (w265:dbl[][])
              n100 = Greater?(x=w293, y=w292) -> (0:w291:bool)
              "Read?" <- w291
              n101 = case shown="True" w291 {
                tunnel: [w311 w336] -> w288
                tunnel: w285 -> [w312 w335]
                tunnel: [w312 w315] -> w284
                tunnel: T6 {"Com Port"=1, "ISOBUS Address"=0, "GPIB Address"=25, "Communication"=enum."GPIB"} ("Address") -> [_ w334]
                tunnel: [w310 w330] -> w272
                frame False {
                  n102 = local read "Setpoint Temperature (K)"() -> (w310:dbl)
                  n103 = local read "Actual Temperature (K)"() -> (w311:dbl)
                }
                frame True {
                  w331 = u32 1000 ("byte count")
                  # "Temperature/Magnet read"
                  n104 = local read "Lock_in_Amplifier"() -> (w319:refnum<visa-resource-name>)
                  n105 = local read "Lake Shore"() -> (w333:refnum<visa-resource-name>)
                  n106 = local read "Magnet"() -> (w322:bool)
                  n107 = case shown="True" w322 {
                    tunnel: w334 -> [_ w340]
                    frame False {
                    }
                    frame True {
                      n108 = call "GPIB - BusCommand.vi"("Command"="R7" ("format string"), "Address"=w340) -> ("Reply"=w341:string)  [unwired: 1 out]
                      n109 = Scan From String(format string="R%f" ("remaining string"), input string=w341) -> (output 1=w339:dbl)  [unwired: 3 in, 3 out]
                      n110 = local write "Nominal Field (T)"(w339) -> ()
                    }
                  }
                  n111 = VISA Write(VISA resource name=w333, write buffer="KRDG?a", error in (no error)=w335) -> (VISA resource name out=w329:refnum<visa-resource-name>, error out=w327:errorcluster)  [unwired: 1 out]
                  n112 = VISA Read(VISA resource name=w329, byte count=w331, error in (no error)=w327) -> (VISA resource name out=w328:refnum<visa-resource-name>, read buffer=w337:string, error out=w326:errorcluster)  [unwired: 1 out]
                  n113 = VISA Write(VISA resource name=w328, write buffer="SETP?a", error in (no error)=w326) -> (VISA resource name out=w324:refnum<visa-resource-name>, error out=w325:errorcluster)  [unwired: 1 out]
                  n114 = Fract/Exp String To Number(string=w337) -> (number=w336:dbl)  [unwired: 3 in, 1 out]
                  n115 = VISA Read(VISA resource name=w324, byte count=w331, error in (no error)=w325) -> (read buffer=w323:string, error out=w321:errorcluster)  [unwired: 2 out]
                  n116 = VISA Write(VISA resource name=w319, write buffer="OUTP? 3", error in (no error)=w321) -> (VISA resource name out=w318:refnum<visa-resource-name>, error out=w320:errorcluster)  [unwired: 1 out]
                  n117 = VISA Read(VISA resource name=w318, byte count=u32 1000, error in (no error)=w320) -> (read buffer=w314:string, error out=w315:errorcluster)  [unwired: 2 out]
                  n118 = Fract/Exp String To Number(string=w314) -> (number=→"LockInR":dbl)  [unwired: 3 in, 1 out]
                  n119 = Fract/Exp String To Number(string=w323) -> (number=w330:dbl)  [unwired: 3 in, 1 out]
                }
              }
              "Actual Temperature (K)" <- w288
              "Setpoint Temperature (K)" <- w272
              n120 = Index Array(array=w265, index (row)=0) -> (element=w261:dbl[])  [unwired: 1 in]
              n121 = Index Array(array=w265, index (row)=1 ("index (col)")) -> (element=w264:dbl[])  [unwired: 1 in]
              n122 = Threshold 1D Array(2:w263, 3:w264) -> (0:w262:dbl)  [unwired: 1 in]
              n123 = Interpolate 1D Array(1:w262, 2:w261) -> (0:w260:dbl)
              "Actual B Field (T)" <- w260
              n124 = Build Array (concatenate)(w295, w260) -> (w296:dbl[])
              "Magnetic Field (T)" <- w296
              n125 = Build Array (concatenate)(w290, w288) -> (w289:dbl[])
              "Temperature array" <- w289
              n126 = case shown="True" "Sweep" {
                tunnel: [Mode."Plot" ("Enum") Mode."Sweep" ("Enum")] -> w287
                frame False {
                }
                frame True {
                }
              }
            }
            frame "Sweep" {
              n127 = local read "Temp/Magnetic Field"() -> (w345:bool)
              n128 = case shown="True" w345 {
                tunnel: w355 -> [w364 w421]
                tunnel: [w363 w420] -> w354
                frame False {
                  n129 = local read "Nominal Field (T)"() -> (w359:dbl)
                  n130 = local read "Min Field (T)"() -> (w358:dbl)
                  n131 = local read "Max Field (T)"() -> (w365:dbl)
                  n132 = local read "Read?"() -> (w362:bool)
                  n133 = Greater Or Equal?(x=w358, y=w359) -> (x >= y?=w361:bool)
                  n134 = Compound Arithmetic op=AND(w361, w362) -> (w360:bool)
                  n135 = case shown="False" w360 {
                    tunnel: [w368 w404] -> w363
                    tunnel: w365 -> [w366 w403]
                    tunnel: w358 -> [_ w402]
                    tunnel: w359 -> [_ w400]
                    tunnel: w364 -> [w369 w399]
                    frame True {
                      # "Ramp Up"
                      n136 = case shown="True" "First?" {
                        tunnel: [TRUE ("Save") FALSE ("Save")] -> w372
                        tunnel: [w391 w395] -> w371
                        frame False {
                          n137 = local read "Counter"() -> (w394:i8)
                          n138 = local write "Actual Polarization"(0.0 ("Actual Polarization")) -> ()
                          n139 = Increment(x=w394) -> (x+1=w391:i8)
                          n140 = local write "Counter"(w391) -> ()
                        }
                        frame True {
                          n141 = local read "Counter"() -> (w395:i8)
                          n142 = local write "First?"(FALSE ("First?")) -> ()
                        }
                      }
                      "Reset" <- w372
                      n143 = local write "Read?"(FALSE ("Read?")) -> ()
                      n144 = local read "Record ALL"() -> (w367:bool)
                      n145 = case shown="True" w367 {
                        tunnel: w371 -> [_ w379]
                        tunnel: [FALSE w377] -> w370
                        frame False {
                        }
                        frame True {
                          n146 = Greater?(x=w379, y="Max Countl") -> (0:w377:bool)
                        }
                      }
                      n147 = case shown="True" w370 {
                        tunnel: w369 -> [w383 w390]
                        tunnel: [w382 w390] -> w368
                        tunnel: w366 -> [w381 _]
                        frame False {
                          n148 = local read "Magnet"() -> (w380:bool)
                          n149 = case shown="True" w380 {
                            tunnel: w383 -> [w384 w387]
                            tunnel: [w384 w386] -> w382
                            tunnel: w381 -> [_ w385]
                            frame False {
                            }
                            frame True {
                              n150 = call "Set_B.vi"("error in (no error)"=w387, "address string"="25", "Set Field (T)"=w385) -> ("error out"=w386:errorcluster)  [unwired: 8 in]
                            }
                          }
                          "Target Field" <- w381
                        }
                        frame True {
                          "New" <- TRUE
                        }
                      }
                      "Up/Down" <- FALSE ("Up/Down")
                    }
                    frame False {
                      n151 = Less Or Equal?(x=w403, y=w400) -> (x <= y?=w401:bool)
                      n152 = case shown="True" w401 {
                        tunnel: [w405 w409] -> w404
                        tunnel: w402 -> [_ w407]
                        tunnel: w399 -> [w405 w410]
                        frame False {
                        }
                        frame True {
                          # "Resetting at the end of every cycle"
                          # "Ramp Dn"
                          n153 = local write "Up/Down"(TRUE ("Up/Down")) -> ()
                          n154 = local read "Magnet"() -> (w406:bool)
                          n155 = local write "Target Field"(w407) -> ()
                          n156 = local write "Reset"(TRUE ("Reset")) -> ()
                          n157 = case shown="True" w406 {
                            tunnel: w410 -> [w412 w415]
                            tunnel: [w412 w414] -> w409
                            tunnel: w407 -> [_ w413]
                            frame False {
                            }
                            frame True {
                              n158 = call "Set_B.vi"("error in (no error)"=w415, "address string"="25", "Set Field (T)"=w413) -> ("error out"=w414:errorcluster)  [unwired: 8 in]
                            }
                          }
                        }
                      }
                      n159 = local write "Read?"(FALSE ("Read?")) -> ()
                    }
                  }
                }
                frame True {
                  n160 = local read "Setpoint Temperature (K)"() -> (w419:dbl)
                  n161 = local read "Min Temperature (K)"() -> (w418:dbl)
                  n162 = local read "Read?"() -> (w424:bool)
                  n163 = local read "Max temperature (K)"() -> (w417:dbl)
                  n164 = Equal?(x=w419, y=w418) -> (x = y?=w422:bool)
                  n165 = And(x=w422, y=w424) -> (x .and. y?=w423:bool)
                  n166 = case shown="True" w423 {
                    tunnel: [w425 w462] -> w420
                    tunnel: w417 -> [w433 w461]
                    tunnel: w418 -> [_ w460]
                    tunnel: w419 -> [_ w458]
                    tunnel: w421 -> [w426 w457]
                    frame True {
                      # "Ramp Up"
                      n167 = local read "First?"() -> (w437:bool)
                      n168 = case shown="False" w437 {
                        tunnel: [TRUE ("Save") FALSE ("Save")] -> w428
                        tunnel: [w449 w455] -> w431
                        frame False {
                          n169 = local read "Counter"() -> (w452:i8)
                          n170 = local write "Actual Polarization"(0.0 ("Actual Polarization")) -> ()
                          n171 = Increment(x=w452) -> (x+1=w449:i8)
                          n172 = local write "Counter"(w449) -> ()
                        }
                        frame True {
                          n173 = local read "Counter"() -> (w455:i8)
                          n174 = local write "First?"(FALSE ("First?")) -> ()
                        }
                      }
                      n175 = local write "Read?"(FALSE ("Read?")) -> ()
                      n176 = Number To Fractional String(number=w433, precision (6)=i16 3) -> (F-format string=w435:string)  [unwired: 2 in]
                      n177 = local read "Record ALL"() -> (w432:bool)
                      n178 = Concatenate Strings("SETP 1," ("write buffer"), w435) -> (w427:string)
                      n179 = case shown="True" w432 {
                        tunnel: w431 -> [_ w448]
                        tunnel: [FALSE w447] -> w429
                        frame False {
                        }
                        frame True {
                          n180 = local read "Max Countl"() -> (w446:i32)
                          n181 = Greater?(x=w448, y=w446) -> (0:w447:bool)
                        }
                      }
                      n182 = local write "Reset"(w428) -> ()
                      n183 = case shown="True" w429 {
                        tunnel: w427 -> [w442 _]
                        tunnel: w426 -> [w440 w443]
                        tunnel: [w439 w443] -> w425
                        frame False {
                          n184 = local read "Lake Shore"() -> (w441:refnum<visa-resource-name>)
                          n185 = VISA Write(VISA resource name=w441, write buffer=w442, error in (no error)=w440) -> (error out=w439:errorcluster)  [unwired: 2 out]
                        }
                        frame True {
                          n186 = local write "New"(TRUE ("New")) -> ()
                        }
                      }
                      "Up/Down 2" <- FALSE ("Up/Down")
                    }
                    frame False {
                      n187 = Equal?(x=w461, y=w458) -> (x = y?=w459:bool)
                      n188 = case shown="True" w459 {
                        tunnel: [w463 w467] -> w462
                        tunnel: w460 -> [_ w466]
                        tunnel: w457 -> [w463 w468]
                        frame False {
                        }
                        frame True {
                          w464 = TRUE ("Reset")
                          # "Ramp Dn"
                          n189 = local write "Up/Down 2"(w464) -> ()
                          n190 = Number To Fractional String(number=w466, precision (6)=i16 3) -> (F-format string=w470:string)  [unwired: 2 in]
                          n191 = local write "Reset"(w464) -> ()
                          n192 = local read "Lake Shore"() -> (w465:refnum<visa-resource-name>)
                          n193 = Concatenate Strings("SETP 1," ("write buffer"), w470) -> (w472:string)
                          n194 = VISA Write(VISA resource name=w465, write buffer=w472, error in (no error)=w468) -> (error out=w467:errorcluster)  [unwired: 2 out]
                        }
                      }
                      n195 = local write "Read?"(FALSE ("Read?")) -> ()
                    }
                  }
                }
              }
              n196 = local read "Magnet"() -> (w344:bool)
              n197 = case shown="False" w344 {
                tunnel: [Mode."StepDelta" ("Enum") Mode."Plot" ("Enum")] -> w346
                frame False {
                }
                frame True {
                }
              }
            }
            frame "StepDelta" {
              n198 = flat-sequence {
                tunnel: w474 -> [w489]
                tunnel: [w488] -> w473
                frame #0 {
                  # "Check if it is time to step Field"
                  n199 = local read "Sweep Rate (T/min)"() -> (w490:dbl)
                  n200 = local read "Time Lag"() -> (w486:dbl)
                  n201 = xnode "Sweep Delay"("SweepRate"=w490, "Resolution"=0.001 ("Voltage Step (V)")) -> ("Result"=w487:dbl)  [unwired: 2 in, 1 out]
                  n202 = Divide(x=w486, y=w487) -> (x/y=w484:dbl)
                  n203 = Multiply(x=0.001 ("y"), y=w484) -> (x*y=w483:dbl)
                  "deltaUaux" <- w483
                  n204 = stacked-sequence {
                    tunnel: w489 -> [_ w501]
                    tunnel: [_ w500] -> w488
                    tunnel: w483 -> [w495 _]
                    frame #0 {
                      n205 = local read "Hall Resistance (Ohm)"() -> (w498:dbl)
                      n206 = local read "Up/Down"() -> (w499:bool)
                      n207 = Add(x=w498, y=w495) -> (x+y=w497:dbl)
                      n208 = Subtract(x=w498, y=w495) -> (x-y=w496:dbl)
                      n209 = local read "Calibration Curve Data"() -> (w494:dbl[][])
                      n210 = Select(t=w496, s=w499, f=w497) -> (s? t:f=w492:dbl)
                      "Hall Resistance (Ohm)" <- w492
                      n211 = call "HallR_to_B.vi"("Measured R(Ohm)"=w492, "Calibration Curve Data"=w494) -> ("Interpolated B value"=w493:dbl)  [unwired: 9 in]
                      n212 = local write "Nominal Field (T)"(w493) -> ()
                    }
                    frame #1 {
                      n213 = local read "Hall Resistance (Ohm)"() -> (w506:dbl)
                      n214 = local read "Lock_in_Amplifier"() -> (w502:refnum<visa-resource-name>)
                      n215 = Format Into String(w506) -> (resulting string=w505:string)  [unwired: 3 in, 1 out]
                      n216 = Concatenate Strings("AUXV 1,", w505) -> (w503:string)
                      n217 = VISA Write(VISA resource name=w502, write buffer=w503, error in (no error)=w501) -> (error out=w500:errorcluster)  [unwired: 2 out]
                    }
                  }
                }
              }
            }
            frame "Plot" {
              # "dI"
              n218 = local read "Nominal Field (T)"() -> (w526:dbl)
              n219 = local read "Actual B Field (T)"() -> (w525:dbl)
              n220 = local read "P(uC/mm^2)"() -> (w528:dbl[])
              n221 = local read "B lag"() -> (w521:cluster{dbl[], dbl[]})
              n222 = local read "Actual Polarization"() -> (w527:dbl)
              n223 = Unbundle(w521) -> (w520:dbl[], w519:dbl[])
              n224 = Build Array (concatenate)(w519, w525) -> (w523:dbl[])
              n225 = Build Array (concatenate)(w520, w526) -> (w524:dbl[])
              n226 = local read "Actual Current (pA)"() -> (w529:dbl)
              n227 = local read "Time Lag"() -> (w541:dbl)
              n228 = Bundle(w524, w523) -> (→"B lag":cluster{dbl[], dbl[]})  [unwired: 1 in]
              n229 = Multiply(x=w529, y=w541) -> (x*y=w533:dbl)
              n230 = Divide(x=w533, y="Sample area (mm^2)") -> (x/y=w532:dbl)
              n231 = Add(x=w532, y=w527) -> (x+y=w531:dbl)
              "Actual Polarization" <- w531
              n232 = local read "Temp/Magnetic Field"() -> (w542:bool)
              n233 = Build Array (concatenate)(w528, w531) -> (→"P(uC/mm^2)":dbl[])
              n234 = case shown="False" w542 {
                tunnel: w539 -> [_ w602]
                tunnel: w536 -> [_ w584]
                tunnel: w531 -> [w549 w585]
                frame False {
                  # "Magnetic Field plotting"
                  n235 = local read "Up/Down"() -> (w554:bool)
                  n236 = case shown="False" w554 {
                    frame True {
                      # "Down"
                      n237 = local read "I(B) 3"() -> (w564:cluster{dbl[], dbl[]}[])
                      n238 = local read "I(B) 3"() -> (w568:cluster{dbl[], dbl[]}[])
                      n239 = Index Array(array=w564, index=1) -> (element=w562:cluster{dbl[], dbl[]})
                      n240 = Unbundle(w562) -> (w561:dbl[], w560:dbl[])
                      n241 = Index Array(array=w568, index=i8 0 ("t")) -> (element=w565:cluster{dbl[], dbl[]})
                      n242 = local read "Actual Current (pA)"() -> (w555:dbl)
                      n243 = local read "Actual B Field (T)"() -> (w557:dbl)
                      n244 = Build Array (concatenate)(w561, w557) -> (w559:dbl[])
                      n245 = Build Array (concatenate)(w560, w555) -> (w558:dbl[])
                      n246 = Bundle(w559, w558) -> (w556:cluster{dbl[], dbl[]})  [unwired: 1 in]
                      n247 = Build Array(w565, w556) -> (w566:cluster{dbl[], dbl[]}[])
                      n248 = local write "I(B) 3"(w566) -> ()
                    }
                    frame False {
                      # "Up"
                      n249 = local read "I(B) 3"() -> (w580:cluster{dbl[], dbl[]}[])
                      n250 = local read "I(B) 3"() -> (w582:cluster{dbl[], dbl[]}[])
                      n251 = Index Array(array=w580, index=0) -> (element=w578:cluster{dbl[], dbl[]})
                      n252 = Unbundle(w578) -> (w577:dbl[], w576:dbl[])
                      n253 = Index Array(array=w582, index=i8 1 ("t")) -> (element=w571:cluster{dbl[], dbl[]})
                      n254 = local read "Actual B Field (T)"() -> (w572:dbl)
                      n255 = Build Array (concatenate)(w577, w572) -> (w575:dbl[])
                      n256 = local read "Actual Current (pA)"() -> (w569:dbl)
                      n257 = Build Array (concatenate)(w576, w569) -> (w574:dbl[])
                      n258 = Bundle(w575, w574) -> (w573:cluster{dbl[], dbl[]})  [unwired: 1 in]
                      n259 = Build Array(w573, w571) -> (w570:cluster{dbl[], dbl[]}[])
                      n260 = local write "I(B) 3"(w570) -> ()
                    }
                  }
                  n261 = local read "Actual B Field (T)"() -> (w551:dbl)
                  n262 = local read "P(B)"() -> (w553:cluster{"yi":dbl[], dbl[]})
                  n263 = Unbundle(w553) -> ("yi"=w552:dbl[], w550:dbl[])
                  n264 = Build Array (concatenate)(w552, w551) -> (w548:dbl[])
                  n265 = Build Array (concatenate)(w550, w549) -> (w547:dbl[])
                  n266 = Bundle(w548, w547) -> (→"P(B)":cluster{dbl[], dbl[]})  [unwired: 1 in]
                }
                frame True {
                  # "Temperature plotting"
                  n267 = Quotient & Remainder(x=w602, y="Save Period") -> (x-y*floor(x/y)=w583:dbl)  [unwired: 1 out]
                  n268 = Greater?(x=w584, y=w583) -> (0:w600:bool)
                  n269 = local read "Actual Temperature (K)"() -> (w587:dbl)
                  n270 = local read "Actual Current (pA)"() -> (w593:dbl)
                  n271 = local read "P(T)"() -> (w589:cluster{"yi":dbl[], dbl[]})
                  n272 = local read "I(T)"() -> (w599:cluster{dbl[], dbl[]})
                  n273 = case shown="True" w600 {
                    frame False {
                    }
                    frame True {
                      n274 = local write "Reset"(TRUE) -> ()
                    }
                  }
                  n275 = Unbundle(w589) -> ("yi"=w590:dbl[], w586:dbl[])
                  n276 = Unbundle(w599) -> (w597:dbl[], w596:dbl[])
                  n277 = Build Array (concatenate)(w590, w587) -> (w591:dbl[])
                  n278 = Build Array (concatenate)(w586, w585) -> (w592:dbl[])
                  n279 = Build Array (concatenate)(w597, w587) -> (w595:dbl[])
                  n280 = Build Array (concatenate)(w596, w593) -> (w594:dbl[])
                  n281 = Bundle(w595, w594) -> (→"I(T)":cluster{dbl[], dbl[]})  [unwired: 1 in]
                  n282 = Bundle(w591, w592) -> (→"P(T)":cluster{dbl[], dbl[]})  [unwired: 1 in]
                }
              }
            }
            frame "Save" {
              n283 = local read "Reset"() -> (w604:bool)
              n284 = case shown="True" w604 {
                tunnel: w609 -> [w626 w628]
                tunnel: [w626 w631] -> w614
                tunnel: w608 -> [w625 w629]
                tunnel: [w625 w631] -> w613
                tunnel: w610 -> [w624 w630]
                tunnel: [w624 w631] -> w612
                tunnel: [w623 w631] -> w611
                tunnel: w607 -> [w623 w627]
                frame False {
                }
                frame True {
                  n285 = stacked-sequence {
                    tunnel: [_ _ w713] -> w631
                    tunnel: w630 -> [_ w702 _]
                    tunnel: w629 -> [w634 w700 _]
                    tunnel: w628 -> [w635 w701 _]
                    tunnel: w627 -> [w633 w698 _]
                    frame #0 {
                      n286 = local read "Temp/Magnetic Field"() -> (w632:bool)
                      n287 = case shown="True" w632 {
                        tunnel: w635 -> [w662 w689]
                        tunnel: w634 -> [w661 w688]
                        tunnel: w633 -> [w652 w679]
                        frame False {
                          n288 = local read "B array"() -> (w646:dbl[])
                          n289 = local read "Counter"() -> (w660:i8)
                          n290 = local read "Averaged I(B)"() -> (w637:dbl[][])
                          n291 = local read "Up/Down"() -> (w663:bool)
                          n292 = local read "Sample area (mm^2)"() -> (w642:dbl)
                          n293 = call "Average_IBP_curves_baseline.vi"("I in"=w661, "Averaged P(B) In"="Averaged P(B)", "Counter"=w660, "B0"="Threshold B (T)", "Averaged I(B) In"=w637, "t in"=w652, "B in"=w662, "Averaged dt in"="Averaged dt", "Up/Down"=w663, "Sample area(mm^2)"=w642, "B array"=w646) -> ("Averaged dt Out"=w649:dbl[][], "Averaged P(B) Out"=w638:dbl[][], "BaselineSubtracted I(B)"=w636:dbl[][])  [unwired: 1 in, 1 out]
                          "Averaged I(B)" <- w636
                          n294 = Index Array(array=w638, index (row)=0 ("disabled index (col)")) -> (element=w647:dbl[])  [unwired: 1 in]
                          n295 = Index Array(array=w638, index (row)=1 ("disabled index (col)")) -> (element=w648:dbl[])  [unwired: 1 in]
                          n296 = Index Array(array=w636, index (row)=0 ("disabled index (col)")) -> (element=w654:dbl[])  [unwired: 1 in]
                          n297 = Index Array(array=w636, index (row)=1 ("disabled index (col)")) -> (element=w653:dbl[])  [unwired: 1 in]
                          n298 = local write "Averaged dt"(w649) -> ()
                          n299 = Bundle("B array"=w646, "Averaged P(B) Out"=w647) -> (w645:T7)  [unwired: 1 in]
                          n300 = Bundle("B array"=w646, "Averaged P(B) Out"=w648) -> (w644:T7)  [unwired: 1 in]
                          n301 = local write "Averaged P(B)"(w638) -> ()
                          n302 = Bundle("B array"=w646, "BaselineSubtracted I(B)"=w654) -> (w659:T8)  [unwired: 1 in]
                          n303 = Bundle("B array"=w646, "BaselineSubtracted I(B)"=w653) -> (w658:T8)  [unwired: 1 in]
                          n304 = Build Array(w645, w644) -> (→"P(B) /Averaged/":T9)
                          n305 = Build Array(w659, w658) -> (→"I(B) /Averaged/":T10)
                        }
                        frame True {
                          n306 = local read "T array"() -> (w674:dbl[])
                          n307 = local read "Counter"() -> (w687:i8)
                          n308 = local read "Averaged I(T)"() -> (w666:dbl[][])
                          n309 = local read "Up/Down"() -> (w690:bool)
                          n310 = local read "Averaged dt"() -> (w665:dbl[][])
                          n311 = local read "Sample area (mm^2)"() -> (w670:dbl)
                          n312 = call "Average_ITP_curves.vi"("I in"=w688, "Averaged P(T) In"="Averaged P(T)", "Counter"=w687, "Averaged I(T) In"=w666, "t in"=w679, "T in"=w689, "Averaged dt in"=w665, "Up/Down"=w690, "Sample area(mm^2)"=w670, "T array"=w674) -> ("Averaged I(B) out"=w664:dbl[][], "Averaged dt Out"=w677:dbl[][], "Averaged P(T) Out"=w667:dbl[][])  [unwired: 3 in]
                          "Averaged I(T)" <- w664
                          n313 = Index Array(array=w667, index (row)=0 ("disabled index (col)")) -> (element=w675:dbl[])  [unwired: 1 in]
                          n314 = Index Array(array=w667, index (row)=1 ("disabled index (col)")) -> (element=w676:dbl[])  [unwired: 1 in]
                          n315 = Index Array(array=w664, index (row)=0 ("disabled index (col)")) -> (element=w681:dbl[])  [unwired: 1 in]
                          n316 = Index Array(array=w664, index (row)=1 ("disabled index (col)")) -> (element=w680:dbl[])  [unwired: 1 in]
                          n317 = local write "Averaged dt"(w677) -> ()
                          n318 = Bundle("T array"=w674, "Averaged P(T) Out"=w675) -> (w673:T11)  [unwired: 1 in]
                          n319 = Bundle("T array"=w674, "Averaged P(T) Out"=w676) -> (w672:T11)  [unwired: 1 in]
                          n320 = local write "Averaged P(T)"(w667) -> ()
                          n321 = Bundle("T array"=w674, "Averaged I(B) out"=w681) -> (w686:T12)  [unwired: 1 in]
                          n322 = Bundle("T array"=w674, "Averaged I(B) out"=w680) -> (w685:T12)  [unwired: 1 in]
                          n323 = Build Array(w673, w672) -> (→"P(T) /Averaged/":T13)
                          n324 = Build Array(w686, w685) -> (→"I(T) /Averaged/":T14)
                        }
                      }
                    }
                    frame #1 {
                      # "Save and Reset"
                      n325 = local read "Sweep"() -> (w691:bool)
                      n326 = local read "Measurement File"() -> (w693:path)
                      n327 = local read "P(uC/mm^2)"() -> (w699:dbl[])
                      n328 = Build Array(w702, w701, w700, w698, w699) -> (w692:dbl[][])
                      n329 = case shown="True" w691 {
                        tunnel: w692 -> [_ w709]
                        frame False {
                        }
                        frame True {
                          n330 = local read "Up/Down"() -> (w705:bool)
                          n331 = case shown="True" w705 {
                            tunnel: [w710 w711] -> w704
                            frame False {
                              n332 = local read "Measurement File_dn"() -> (w710:path)
                            }
                            frame True {
                              n333 = local read "Measurement File_up"() -> (w711:path)
                            }
                          }
                          n334 = call-poly <vilib>:"Write Delimited Spreadsheet.vi"("file path (dialog if empty)"=w704, "format (%.3f)"="%.5g", "2D data"=w709, "append to file? (F)"=TRUE ("transpose? (F)"), "transpose? (F)"=FALSE ("append to file? (F)")) -> ()  [unwired: 9 in, 2 out]
                        }
                      }
                      n335 = case shown="False" "Reset IB?" {
                        frame False {
                        }
                        frame True {
                          n336 = local read "Up/Down"() -> (w712:bool)
                          n337 = case shown="False" w712 {
                            frame False {
                              n338 = invoke on="I(B) 3" class="XYGraph (strict)" method="Reinit To Default"() -> ()  [unwired: 3 in, 3 out]
                              n339 = invoke on="I(T)" class="XYGraph (strict)" method="Reinit To Default"() -> ()  [unwired: 3 in, 3 out]
                            }
                            frame True {
                            }
                          }
                        }
                      }
                      n340 = call-poly <vilib>:"Write Delimited Spreadsheet.vi"("file path (dialog if empty)"=w693, "format (%.3f)"="%.5g", "2D data"=w692, "append to file? (F)"=TRUE, "transpose? (F)"=TRUE) -> ()  [unwired: 9 in, 2 out]
                      n341 = local write "Reset"(FALSE ("Save")) -> ()
                    }
                    frame #2 {
                      w713 = dbl[] []
                      n342 = local write "P(uC/mm^2)"(w713) -> ()
                    }
                  }
                }
              }
              n343 = local read "New"() -> (w606:bool)
              n344 = case shown="False" w606 {
                tunnel: [Mode."Return" ("Enum") Mode."New" ("Enum")] -> w618
                tunnel: [TRUE FALSE] -> w605
                frame False {
                }
                frame True {
                }
              }
            }
            frame "New" {
              n345 = stacked-sequence {
                seq-local: [_ _ _ _ w815 _ _] -> [_ _ _ _ _ w824 _]
                seq-local: [_ _ w769 _ _ _ _] -> [_ _ _ _ w814 _ _]
                tunnel: T6 {"Com Port"=1, "ISOBUS Address"=0, "GPIB Address"=25, "Communication"=enum."GPIB"} ("Address") -> [_ _ w768 w809 _ _ _]
                tunnel: w716 -> [_ _ w770 _ _ w825 _]
                tunnel: [_ _ _ _ _ w827 _] -> w715
                tunnel: w714 -> [_ w749 _ _ _ _ _]
                frame #0 {
                  w742 = 1 ("index (row)")
                  w741 = 0 ("index (row)")
                  # "Save averages"
                  n346 = local read "Measurement File_average"() -> (w729:path)
                  n347 = local read "Averaged P(B)"() -> (w740:dbl[][])
                  n348 = local read "Averaged dt"() -> (w738:dbl[][])
                  n349 = local read "I(B) /Averaged/"() -> (w730:cluster{"B array":dbl[], dbl[]}[])
                  n350 = Index Array(array=w738, index (row)=w741) -> (element=w739:dbl[])  [unwired: 1 in]
                  n351 = Index Array(array=w738, index (row)=w742) -> (element=w746:dbl[])  [unwired: 1 in]
                  n352 = Index Array(array=w730, index=1) -> (element=w734:cluster{"B array":dbl[], dbl[]})
                  n353 = Index Array(array=w730, index=0) -> (element=w733:cluster{"B array":dbl[], dbl[]})
                  n354 = Unbundle(w734) -> ("B array"=w744:dbl[], w745:dbl[])
                  n355 = Unbundle(w733) -> ("B array"=w735:dbl[], w736:dbl[])
                  n356 = Index Array(array=w740, index (row)=w741) -> (element=w743:dbl[])  [unwired: 1 in]
                  n357 = Index Array(array=w740, index (row)=w742) -> (element=w747:dbl[])  [unwired: 1 in]
                  n358 = Build Array(w735, w736, w739, w743, w744, w745, w746, w747) -> (w737:dbl[][])
                  n359 = call-poly <vilib>:"Write Delimited Spreadsheet.vi"("file path (dialog if empty)"=w729, "format (%.3f)"="%.5g", "2D data"=w737, "append to file? (F)"=TRUE ("transpose? (F)"), "transpose? (F)"=TRUE ("append to file? (F)")) -> ()  [unwired: 9 in, 2 out]
                }
                frame #1 {
                  w755 = dbl[] []
                  w764 = dbl[] []
                  # "Reset Flags"
                  n360 = Get Date/Time In Seconds() -> (seconds since 1Jan1904=w765:timestamp)
                  n361 = local write "Up/Down"(TRUE ("Up/Down")) -> ()
                  n362 = local write "First?"(TRUE ("First?")) -> ()
                  n363 = local write "Offset?"(FALSE ("Offset?")) -> ()
                  n364 = local write "New"(FALSE ("New")) -> ()
                  n365 = local write "P(uC/mm^2)"(w764) -> ()
                  n366 = local write "Start time"(w765) -> ()
                  n367 = local write "Actual Polarization"(0.0 ("Actual Polarization")) -> ()
                  n368 = local write "Offset array"(w764) -> ()
                  n369 = local write "Up/Down"(TRUE ("Up/Down")) -> ()
                  n370 = local write "Reset"(FALSE ("Reset")) -> ()
                  n371 = local read "B array"() -> (w758:dbl[])
                  n372 = local write "Counter"(i8 0 ("Counter")) -> ()
                  n373 = invoke on="P(B)" class="XYGraph (strict)" method="Reinit To Default"() -> ()  [unwired: 3 in, 3 out]
                  n374 = invoke on="I(B) 3" class="XYGraph (strict)" method="Reinit To Default"() -> ()  [unwired: 3 in, 3 out]
                  n375 = Multiply(x=w758, y=0.0) -> (x*y=w759:dbl[])
                  n376 = Build Array(w755, w755) -> (w763:dbl[][])
                  n377 = Bundle("B array"=w758, w759) -> (w760:cluster{"B array":dbl[], dbl[]})  [unwired: 1 in]
                  n378 = local write "Averaged I(B)"(w763) -> ()
                  n379 = Build Array(w760, w760) -> (w761:cluster{"B array":dbl[], dbl[]}[])
                  n380 = local write "I(B) /Averaged/"(w761) -> ()
                  n381 = local write "Measuring"(FALSE ("Measuring")) -> ()
                  n382 = Flush Queue(queue=w749) -> (remaining elements=→"remaining elements 2":T1)  [unwired: 1 in, 2 out]
                }
                frame #2 {
                  # "Step"
                  n383 = local read "Sweep Rate Array"() -> (w774:dbl[])
                  n384 = local read "j"() -> (w775:i32)
                  n385 = Increment(x=w775) -> (x+1=w771:i32)
                  n386 = Array Size(array=w774) -> (size(s)=w773:i32)
                  n387 = Less?(x=w771, y=w773) -> (x < y?=w772:bool)
                  "Step Rate" <- w772
                  n388 = case shown="True" w772 {
                    tunnel: w771 -> [_ w802]
                    tunnel: w770 -> [w778 w801]
                    tunnel: [w777 w801] -> w769
                    tunnel: w768 -> [w776 _]
                    frame False {
                      # "Step Temp?"
                      n389 = local read "Temperature Array"() -> (w782:dbl[])
                      n390 = local read "i"() -> (w783:i32)
                      n391 = Increment(x=w783) -> (x+1=w780:i32)
                      n392 = local write "j"(0 ("f")) -> ()
                      n393 = Array Size(array=w782) -> (size(s)=w781:i32)
                      n394 = Less?(x=w780, y=w781) -> (x < y?=w779:bool)
                      "Step Temp" <- w779
                      n395 = case shown="False" w779 {
                        tunnel: w780 -> [_ w800]
                        tunnel: w778 -> [w788 w799]
                        tunnel: [w787 w799] -> w777
                        tunnel: w776 -> [w786 _]
                        frame False {
                          # "Heater OFF"
                          # "Finished"
                          n396 = local write "i"(0 ("i")) -> ()
                          n397 = stacked-sequence {
                            tunnel: w788 -> [w792 _ _]
                            tunnel: [w791 _ _] -> w787
                            tunnel: w786 -> [_ w796 w797]
                            frame #0 {
                              n398 = local read "Lake Shore"() -> (w793:refnum<visa-resource-name>)
                              n399 = VISA Write(VISA resource name=w793, write buffer="RANGE,1,0", error in (no error)=w792) -> (error out=w791:errorcluster)  [unwired: 2 out]
                            }
                            frame #1 {
                              n400 = call "ips_switchHeaterOff.vi"("Instrument address"=w796, "Rate"=2.0) -> ()  [unwired: 1 out]
                            }
                            frame #2 {
                              n401 = call "GPIB - BusCommand.vi"("Command"="H0", "Address"=w797) -> ()  [unwired: 2 out]
                            }
                          }
                          n402 = local write "Record ALL"(FALSE ("Record ALL")) -> ()
                          "Finished" <- TRUE
                        }
                        frame True {
                          n403 = local write "i"(w800) -> ()
                        }
                      }
                    }
                    frame True {
                      n404 = local write "j"(w802) -> ()
                    }
                  }
                }
                frame #3 {
                  # "Set rates"
                  n405 = local read "Sweep Rate Array"() -> (w808:dbl[])
                  n406 = local read "j"() -> (w807:i32)
                  n407 = local read "j"() -> (w805:i32)
                  n408 = Index Array(array=w808, index=w807) -> (element=w806:dbl)
                  n409 = Number To Fractional String(number=w806, precision (6)=i16 3) -> (F-format string=w812:string)  [unwired: 2 in]
                  n410 = Index Array(array="Max count array", index=w805) -> (element=w803:i32)
                  n411 = local write "Max Countl"(w803) -> ()
                  n412 = Concatenate Strings("T" ("format string"), w812) -> (w813:string)
                  n413 = call "GPIB - BusCommand.vi"("Command"=w813, "Address"=w809) -> ()  [unwired: 2 out]
                  n414 = local write "Sweep Rate (T/min)"(w806) -> ()
                }
                frame #4 {
                  # "Set temperature"
                  n415 = local read "Temperature Array"() -> (w818:dbl[])
                  n416 = local read "i"() -> (w817:i32)
                  n417 = Index Array(array=w818, index=w817) -> (element=w816:dbl)
                  n418 = local read "Lake Shore"() -> (w820:refnum<visa-resource-name>)
                  n419 = Number To Fractional String(number=w816, precision (6)=i16 3) -> (F-format string=w821:string)  [unwired: 2 in]
                  n420 = Concatenate Strings("SETP 1," ("write buffer"), w821) -> (w823:string)
                  n421 = VISA Write(VISA resource name=w820, write buffer=w823, error in (no error)=w814) -> (error out=w815:errorcluster)  [unwired: 2 out]
                }
                frame #5 {
                  n422 = local read "Finished"() -> (w826:bool)
                  n423 = case shown="False" w826 {
                    tunnel: [w840 w879] -> w827
                    tunnel: w825 -> [_ _]
                    tunnel: w824 -> [w837 w879]
                    frame False {
                      w835 = "_" ("string")
                      # "Wait, create Files"
                      n424 = local read "Temperature Array"() -> (w867:dbl[])
                      n425 = local read "Sweep Rate Array"() -> (w863:dbl[])
                      n426 = local read "i"() -> (w866:i32)
                      n427 = local read "j"() -> (w864:i32)
                      n428 = Index Array(array=w867, index=w866) -> (element=w865:dbl)
                      n429 = Index Array(array=w863, index=w864) -> (element=w832:dbl)
                      n430 = Round Toward -Infinity(1:w832) -> (0:w833:dbl)
                      n431 = Number To Fractional String(use system decimal point (T)=TRUE, number=w865, precision (6)=i16 1) -> (F-format string=w868:string)  [unwired: 1 in]
                      n432 = Subtract(x=w832, y=w833) -> (x-y=w834:dbl)
                      n433 = Equal To 0?(x=w834) -> (x = 0?=w831:bool)
                      n434 = Select(t=i16 0 ("precision (6)"), s=w831, f=i16 2 ("precision (6)")) -> (s? t:f=w828:i16)
                      n435 = Number To Fractional String(use system decimal point (T)=TRUE, number=w832, precision (6)=w828) -> (F-format string=w836:string)  [unwired: 1 in]
                      n436 = Concatenate Strings("Directory", "\\" ("string"), "FileName", w835, w868, "K" ("string"), w835, w836, "Tpm" ("string")) -> (w857:string)
                      n437 = local read "Step Temp"() -> (w841:bool)
                      n438 = Search and Replace String(replace all?=TRUE ("replace all? (F)"), input string=w857, search string=".", replace string="p" ("substring (\"\")"), error in=w837) -> (result string=w852:string, error out=w847:errorcluster)  [unwired: 3 in, 2 out]
                      n439 = local write "Step Rate"(FALSE ("Step Rate")) -> ()
                      n440 = Concatenate Strings(w852, ".txt" ("string")) -> (w851:string)
                      n441 = String To Path(string=w851) -> (path=w850:path)
                      n442 = case shown="True" w841 {
                        frame False {
                        }
                        frame True {
                          n443 = call "Calibration_Hall_full.vi"() -> ("Calibration Curve"=w870:cluster{dbl[], "Best Linear Fit":dbl[]}[], "Calibration Curve Data"=w871:dbl[][])  [unwired: 10 in]
                          n444 = local write "Step Temp"(FALSE ("Step Temp")) -> ()
                          n445 = Get Date/Time In Seconds() -> (seconds since 1Jan1904=w872:timestamp)
                          n446 = local write "Calibration Curve Data"(w871) -> ()
                          n447 = local write "Calibration Curve"(w870) -> ()
                          n448 = while {
                            tunnel: w872 -> [w877]
                            stop <- w874 stop-if-true
                            n449 = Get Date/Time In Seconds() -> (seconds since 1Jan1904=w878:timestamp)
                            n450 = Subtract(x=w878, y=w877) -> (x-y=w876:dbl)
                            "Wait (s)" <- w876
                            n451 = Greater Or Equal?(x=w876, y="secs to wait") -> (x >= y?=w874:bool)
                          }
                        }
                      }
                      n452 = Open/Create/Replace File(file path (use dialog)=w850, error in=w847, operation (0:open)=T5."open or create") -> (refnum out=w839:refnum<file>, error out=w840:errorcluster)  [unwired: 3 in, 1 out]
                      n453 = local write "refnum out"(w839) -> ()
                      n454 = Refnum to Path(1:w839) -> (0:w842:path)
                      n455 = call "Create_sweep_files.vi"("Measurement File"=w842) -> ("Path 3"=w845:path, "Path 2"=w844:path, "Path"=w843:path)  [unwired: 8 in]
                      n456 = local write "Measurement File"(w842) -> ()
                      n457 = local write "Measurement File_dn"(w845) -> ()
                      n458 = local write "Measurement File_average"(w843) -> ()
                      n459 = local write "Measurement File_up"(w844) -> ()
                    }
                    frame True {
                    }
                  }
                }
                frame #6 {
                  n460 = local read "Finished"() -> (w880:bool)
                  n461 = case shown="True" w880 {
                    frame False {
                      n462 = local write "Measuring"(TRUE ("Measuring")) -> ()
                    }
                    frame True {
                      n463 = local write "Measure /Pause"(FALSE ("Measure /Pause")) -> ()
                    }
                  }
                }
              }
            }
            frame "Return" {
            }
          }
        }
      }
      frame Error {
        # "Return true for any case which should stop the loop."
      }
    }
  }
  n464 = VISA Read(VISA resource name=w10, byte count=u32 100, error in (no error)=w12) -> (VISA resource name out=w9:refnum<visa-resource-name>, read buffer=w8:string, error out=w11:errorcluster)  [unwired: 1 out]
  n465 = VISA Open(error in (no error)=w11, VISA resource name="Magnetic Field") -> (VISA resource name=w105:refnum<visa-resource-name>, error out=w87:errorcluster)  [unwired: 3 in]
  n466 = VISA Open(error in (no error)=w87, VISA resource name="Lake Shore") -> (VISA resource name=w82:refnum<visa-resource-name>, error out=w51:errorcluster)  [unwired: 3 in]
  n467 = VISA Write(VISA resource name="Lake Shore", write buffer="KRDG?a", error in (no error)=w51) -> (VISA resource name out=w48:refnum<visa-resource-name>, error out=w47:errorcluster)  [unwired: 1 out]
  n468 = VISA Read(VISA resource name=w48, byte count=w54, error in (no error)=w47) -> (VISA resource name out=w45:refnum<visa-resource-name>, read buffer=w59:string, error out=w46:errorcluster)  [unwired: 1 out]
  n469 = VISA Write(VISA resource name=w45, write buffer="SETP?a", error in (no error)=w46) -> (VISA resource name out=w44:refnum<visa-resource-name>, error out=w43:errorcluster)  [unwired: 1 out]
  n470 = VISA Read(VISA resource name=w44, byte count=w54, error in (no error)=w43) -> (VISA resource name out=w41:refnum<visa-resource-name>, read buffer=w58:string, error out=w42:errorcluster)  [unwired: 1 out]
  n471 = VISA Write(VISA resource name=w41, write buffer="RANGE?a", error in (no error)=w42) -> (VISA resource name out=w39:refnum<visa-resource-name>, error out=w40:errorcluster)  [unwired: 1 out]
  n472 = Fract/Exp String To Number(string=w59) -> (number=w57:dbl)  [unwired: 3 in, 1 out]
  n473 = VISA Read(VISA resource name=w39, byte count=w54, error in (no error)=w40) -> (read buffer=w53:string, error out=w50:errorcluster)  [unwired: 2 out]
  n474 = Fract/Exp String To Number(string=w58) -> (number=w56:dbl)  [unwired: 3 in, 1 out]
  n475 = Fract/Exp String To Number(string=w53) -> (number=w49:dbl)  [unwired: 3 in, 1 out]
  n476 = local write "Actual Temperature (K)"(w57) -> ()
  n477 = local write "Setpoint Temperature (K)"(w56) -> ()
  n478 = local write "Heater Range"(w49) -> ()
  n479 = case shown="True" w64 {
    frame False {
    }
    frame True {
      n480 = invoke on="P(T)" class="XYGraph (strict)" method="Reinit To Default"() -> ()  [unwired: 3 in, 3 out]
      n481 = invoke on="I(T)" class="XYGraph (strict)" method="Reinit To Default"() -> ()  [unwired: 3 in, 3 out]
    }
  }
  n482 = Decimal String To Number(string=w8) -> (number=w7:i32)  [unwired: 2 in, 1 out]
  n483 = local write "Keithley (IV conv) averaging"(w7) -> ()
  n484 = while {
    shift-right: [w911] -> w103
    shift-left: w84 -> [w912]
    shift-right: [w913] -> w108
    shift-left: w109 -> [w914]
    tunnel: w9 -> [w910]
    tunnel: w105 -> [w909]
    tunnel: w50 -> [_]
    tunnel: [w903] -> _
    tunnel: w92 -> [w902]
    tunnel: w82 -> [w901]
    tunnel: w17 -> [w900]
    stop <- "stop" stop-if-true
    n485 = event shown="[10] \"Calibrate\": Value Change" {
      selector: _ -> [_ _ _ _ _ _ _ _ _ _ _ _ _ _ _ _]
      dyn-events: _ -> [_ _ _ _ _ _ _ _ _ _ _ _ _ _ _ _]
      timeout: 10 -> [_ _ _ _ _ _ _ _ _ _ _ _ _ _ _ _]
      tunnel: w914 -> [w924 w970 w988 w998 w1012 w1068 w1072 w1076 w1114 w1130 w1147 w1175 w1192 w1208 w1218 w1229]
      tunnel: [w923 w970 w988 w998 w1012 w1068 w1072 w1076 w1114 w1130 w1147 w1175 w1192 w1208 w1218 w1229] -> w913
      tunnel: w912 -> [w922 w979 w987 w997 w1010 w1067 w1074 w1078 w1115 w1129 w1146 w1176 w1194 w1212 w1222 w1231]
      tunnel: [w921 w971 w987 w997 w1009 w1069 w1074 w1077 _ w1129 w1146 w1176 w1193 w1211 w1221 w1230] -> w911
      tunnel: w910 -> [w920 w980 _ _ _ _ _ _ _ _ _ _ _ _ _ _]
      tunnel: w909 -> [w919 _ _ _ _ _ _ _ _ _ _ _ _ _ _ _]
      tunnel: [w917 w969 w986 w996 w1011 w1070 w1073 w1075 w1113 w1128 w1145 w1174 w1191 w1209 w1219 _] -> w903
      tunnel: w902 -> [w917 w969 w986 w999 w1011 w1070 w1073 w1075 w1113 w1128 w1145 w1174 w1191 w1209 w1219 _]
      tunnel: w901 -> [_ _ _ _ _ _ _ _ _ _ _ _ w1195 w1210 w1223 w1228]
      tunnel: [_ _ _ _ _ _ _ _ w1115 _ _ _ _ _ _ _] -> _
      tunnel: w900 -> [w916 _ _ _ _ _ _ _ _ _ _ _ _ _ _ _]
      event Timeout {
        n486 = event-data() -> ()  [unwired: 1 in, 3 out]
        n487 = case shown="True" "Measuring" {
          tunnel: w924 -> [w926 w949]
          tunnel: [w926 w948] -> w923
          tunnel: w922 -> [w925 w927]
          tunnel: [w925 w947] -> w921
          tunnel: w920 -> [_ w940]
          tunnel: w919 -> [_ w939]
          tunnel: w916 -> [_ w930]
          frame False {
          }
          frame True {
            w938 = ":FETCh? " ("data")
            w941 = u32 1000 ("byte count")
            # "Generate the data here."
            n488 = case shown="No Error" w927 {
              selector: w927 -> [w961 w962]
              tunnel: [w961 w962] -> w935
              tunnel: [w960 _] -> w934
              frame No Error {
                n489 = Get Date/Time In Seconds() -> (seconds since 1Jan1904=w960:timestamp)
              }
              frame Error {
              }
            }
            n490 = VISA Write(VISA resource name=w940, write buffer=w938, error in (no error)=w935) -> (VISA resource name out=w946:refnum<visa-resource-name>, error out=w944:errorcluster)  [unwired: 1 out]
            n491 = VISA Write(VISA resource name=w939, write buffer=w938, error in (no error)=w944) -> (VISA resource name out=w945:refnum<visa-resource-name>, error out=w943:errorcluster)  [unwired: 1 out]
            n492 = VISA Read(VISA resource name=w946, byte count=w941, error in (no error)=w943) -> (read buffer=w936:string, error out=w942:errorcluster)  [unwired: 2 out]
            n493 = VISA Read(VISA resource name=w945, byte count=w941, error in (no error)=w942) -> (read buffer=w937:string, error out=w932:errorcluster)  [unwired: 2 out]
            n494 = case shown="False" "DaQ" {
              tunnel: w932 -> [w951 w957]
              tunnel: [w951 w956] -> w931
              tunnel: w930 -> [_ w955]
              tunnel: [0.0 ("Output") w953] -> w928
              frame False {
              }
              frame True {
                n495 = local read "Number of Samples"() -> (w959:i32)
                n496 = call-poly <vilib>:"DAQmx Read.vi"("task/channels in"=w955, "number of samples per channel"=w959, "error in"=w957) -> ("data"=w958:dbl[], "error out"=w956:errorcluster)  [unwired: 10 in, 1 out]
                n497 = call-poly <vilib>:"Mean.vi"("X"=w958) -> ("mean"=w954:dbl)  [unwired: 1 out]
                "Actual mean" <- w954
                n498 = call "N Point Running Average.vi"("n"="Moving average", "Input"=w954) -> ("Output"=w953:dbl)
              }
            }
            n499 = Bundle("seconds since 1Jan1904"=w934, "read buffer"=w936, "read buffer"=w937, "Output"=w928) -> (w933:T4)  [unwired: 1 in]
            n500 = Enqueue Element(queue=w949, element=w933, error in (no error)=w931) -> (queue out=w948:refnum<queue>, error out=w947:errorcluster)  [unwired: 1 in, 1 out]
          }
        }
      }
      event "Keithley (IV conv) averaging": Value Change {
        n501 = event-data() -> ()  [unwired: 1 in, 6 out]
        n502 = Number To Decimal String(number="Keithley (IV conv) averaging") -> (decimal integer string=w977:string)  [unwired: 1 in]
        n503 = Concatenate Strings("VOLTage:DC:AVERage:COUNt " ("write buffer"), w977) -> (w976:string)
        n504 = VISA Write(VISA resource name=w980, write buffer=w976, error in (no error)=w979) -> (VISA resource name out=w975:refnum<visa-resource-name>, error out=w973:errorcluster)  [unwired: 1 out]
        n505 = VISA Write(VISA resource name=w975, write buffer="VOLTage:DC:AVERage:COUNt?", error in (no error)=w973) -> (VISA resource name out=w968:refnum<visa-resource-name>, error out=w972:errorcluster)  [unwired: 1 out]
        n506 = VISA Read(VISA resource name=w968, byte count=u32 100, error in (no error)=w972) -> (read buffer=w966:string, error out=w971:errorcluster)  [unwired: 2 out]
        n507 = Decimal String To Number(string=w966) -> (number=w965:i32)  [unwired: 2 in, 1 out]
        n508 = Equal?(x="Keithley (IV conv) averaging", y=w965) -> (x = y?=→"Confirm":bool)
      }
      event "Max Field (T)": Value Change {
        n509 = event-data() -> ()  [unwired: 1 in, 6 out]
        n510 = Divide(x="Max Field (T)", y="dB (T)") -> (x/y=w983:dbl)
        n511 = for {
          N: w983 -> [_]
          tunnel: "dB (T)" -> [w993]
          tunnel: [w990] -> w982 mode=indexing
          tunnel: "Min Field (T)" -> [w991]
          tunnel: [0.0] -> _ mode=indexing
          i -> [w994]
          n512 = Multiply(x=w994, y=w993) -> (x*y=w992:dbl)
          n513 = Add(x=w992, y=w991) -> (x+y=w990:dbl)
        }
        "B array" <- w982
      }
      event "Sweep Rate (T/min)": Value Change {
        n514 = event-data() -> ("NewVal"=w1000:dbl)  [unwired: 1 in, 5 out]
        n515 = local read "Magnet"() -> (w995:bool)
        n516 = case shown="False" w995 {
          tunnel: w1000 -> [_ w1007]
          tunnel: w999 -> [w1001 w1003]
          tunnel: [w1001 w1002] -> w996
          frame False {
          }
          frame True {
            n517 = Number To Fractional String(number=w1007, precision (6)=i16 3) -> (F-format string=w1005:string)  [unwired: 2 in]
            n518 = Concatenate Strings("T" ("format string"), w1005) -> (w1004:string)
            n519 = call "GPIB - BusCommand.vi"("Command"=w1004, "Address"=w1003) -> ("Address(thru)"=w1002:T6)  [unwired: 1 out]
          }
        }
      }
      event "Field To Zero": Value Change {
        n520 = event-data() -> ()  [unwired: 1 in, 6 out]
        n521 = Two Button Dialog(message="Do you want to switch off the field?", 1:"No" ("F button name (\"Cancel\")"), 2:"Yes" ("T button name (\"OK\")")) -> (T button?=w1016:bool)
        n522 = case shown="True" w1016 {
          tunnel: w1011 -> [_ w1021]
          tunnel: w1010 -> [w1017 w1019]
          tunnel: [w1017 w1018] -> w1009
          frame False {
          }
          frame True {
            n523 = local read "Magnet"() -> (w1020:bool)
            n524 = case shown="False" w1020 {
              tunnel: w1021 -> [_ w1060]
              tunnel: w1019 -> [w1024 w1057]
              tunnel: [w1023 w1057] -> w1018
              frame False {
                n525 = local read "Lock_in_Amplifier"() -> (w1022:refnum<visa-resource-name>)
                n526 = stacked-sequence {
                  seq-local: [w1027 _] -> [_ w1040]
                  seq-local: [w1025 _] -> [_ w1037]
                  tunnel: w1024 -> [w1029 _]
                  tunnel: [_ w1041] -> w1023
                  tunnel: w1022 -> [w1026 w1038]
                  frame #0 {
                    n527 = VISA Write(VISA resource name=w1026, write buffer="AUXV?1", error in (no error)=w1029) -> (VISA resource name out=w1033:refnum<visa-resource-name>, error out=w1028:errorcluster)  [unwired: 1 out]
                    n528 = VISA Read(VISA resource name=w1033, byte count=u32 1000, error in (no error)=w1028) -> (read buffer=w1030:string, error out=w1027:errorcluster)  [unwired: 2 out]
                    n529 = Fract/Exp String To Number(string=w1030) -> (number=w1025:dbl)  [unwired: 3 in, 1 out]
                  }
                  frame #1 {
                    w1044 = 0.001 ("Voltage Step (V)")
                    n530 = local read "Sweep Rate (T/min)"() -> (w1043:dbl)
                    n531 = xnode "Sweep Delay"("SweepRate"=w1043, "Resolution"=w1044) -> ("Result"=w1042:dbl)  [unwired: 2 in, 1 out]
                    n532 = call "Universal_Ramping.vi"("milliseconds to wait"=w1042, "Initial Voltage (V)"=w1037, "error in (no error)"=w1040, "Voltage Step (V)"=w1044, "Final Voltage (V)"=0.0, "VISA resource name"=w1038) -> ("error out"=w1041:errorcluster, "Actual Voltage (V)"=w1034:dbl)  [unwired: 3 in, 1 out]
                    n533 = local read "Calibration Curve Data"() -> (w1036:dbl[][])
                    n534 = local write "Hall Resistance (Ohm)"(w1034) -> ()
                    n535 = call "HallR_to_B.vi"("Measured R(Ohm)"=w1034, "Calibration Curve Data"=w1036) -> ("Interpolated B value"=w1035:dbl)  [unwired: 9 in]
                    n536 = local write "Actual B Field (T)"(w1035) -> ()
                  }
                }
              }
              frame True {
                n537 = local read "Sweep Rate (T/min)"() -> (w1059:dbl)
                n538 = call "ips_switchHeaterOff.vi"("Instrument address"=w1060, "Rate"=w1059) -> ("B"=w1058:dbl)
                n539 = local write "Nominal Field (T)"(w1058) -> ()
              }
            }
          }
        }
      }
      event "Go to Set": Value Change {
        n540 = event-data() -> ()  [unwired: 1 in, 6 out]
        n541 = local read "Lock_in_Amplifier"() -> (w1063:refnum<visa-resource-name>)
        n542 = local read "Sweep Rate (T/min)"() -> (w1065:dbl)
        n543 = local read "Magnet"() -> (w1066:bool)
        n544 = call "Ramp_Field.vi"("Set Field (T) in"="Set Field (T)", "Sweep Rate (T/min)"=w1065, "error in (no error)"=w1067, "Magnet"=w1066, "VISA Refnum in"=w1063) -> ("error out"=w1069:errorcluster, "Actual Voltage (V)"=w1061:dbl, "Set Field (T) out"=w1064:dbl)  [unwired: 4 in]
        n545 = local write "Actual B Field (T)"(w1064) -> ()
        n546 = local write "Hall Resistance (Ohm)"(w1061) -> ()
      }
      event "Measure /Pause": Value Change {
        n547 = event-data() -> ("NewVal"=w1071:bool)  [unwired: 1 in, 5 out]
        n548 = local write "Measuring"(w1071) -> ()
      }
      event "Stop": Value Change {
        n549 = event-data() -> ()  [unwired: 1 in, 6 out]
        n550 = local read "Measuring"() -> (w1079:bool)
        n551 = case shown="True" w1079 {
          tunnel: w1078 -> [w1080 w1083]
          tunnel: [w1080 w1084] -> w1077
          frame False {
          }
          frame True {
            w1089 = FALSE ("Measuring")
            n552 = local read "SaveSweep"() -> (w1090:bool)
            n553 = local write "Measuring"(w1089) -> ()
            n554 = local write "Measure /Pause"(w1089) -> ()
            n555 = local read "Lock_in_Amplifier"() -> (w1085:refnum<visa-resource-name>)
            n556 = case shown="True" w1090 {
              frame False {
              }
              frame True {
                w1096 = 1 ("index (row)")
                w1097 = 0 ("index (row)")
                n557 = local read "Measurement File_average"() -> (w1109:path)
                n558 = local read "Averaged P(B)"() -> (w1098:dbl[][])
                n559 = local read "Averaged dt"() -> (w1100:dbl[][])
                n560 = local read "I(B) /Averaged/"() -> (w1108:cluster{"B array":dbl[], dbl[]}[])
                n561 = Index Array(array=w1100, index (row)=w1097) -> (element=w1099:dbl[])  [unwired: 1 in]
                n562 = Index Array(array=w1100, index (row)=w1096) -> (element=w1092:dbl[])  [unwired: 1 in]
                n563 = Index Array(array=w1108, index=1) -> (element=w1104:cluster{"B array":dbl[], dbl[]})
                n564 = Index Array(array=w1108, index=0) -> (element=w1105:cluster{"B array":dbl[], dbl[]})
                n565 = Unbundle(w1104) -> ("B array"=w1094:dbl[], w1093:dbl[])
                n566 = Unbundle(w1105) -> ("B array"=w1103:dbl[], w1102:dbl[])
                n567 = Index Array(array=w1098, index (row)=w1097) -> (element=w1095:dbl[])  [unwired: 1 in]
                n568 = Index Array(array=w1098, index (row)=w1096) -> (element=w1091:dbl[])  [unwired: 1 in]
                n569 = Build Array(w1103, w1102, w1099, w1095, w1094, w1093, w1092, w1091) -> (w1101:dbl[][])
                n570 = call-poly <vilib>:"Write Delimited Spreadsheet.vi"("file path (dialog if empty)"=w1109, "format (%.3f)"="%.5g", "2D data"=w1101, "append to file? (F)"=TRUE ("transpose? (F)"), "transpose? (F)"=TRUE ("append to file? (F)")) -> ()  [unwired: 9 in, 2 out]
              }
            }
            n571 = local read "Sweep Rate (T/min)"() -> (w1087:dbl)
            n572 = local read "Set Field (T)"() -> (w1088:dbl)
            n573 = local read "Magnet"() -> (w1086:bool)
            n574 = call "Ramp_Field.vi"("Set Field (T) in"=w1088, "Sweep Rate (T/min)"=w1087, "error in (no error)"=w1083, "Magnet"=w1086, "VISA Refnum in"=w1085) -> ("error out"=w1084:errorcluster, "Actual Voltage (V)"=w1081:dbl, "Set Field (T) out"=w1082:dbl)  [unwired: 4 in]
            n575 = local write "Actual B Field (T)"(w1082) -> ()
            n576 = local write "Hall Resistance (Ohm)"(w1081) -> ()
          }
        }
      }
      event "Sweep": Value Change {
        n577 = event-data() -> ("NewVal"=w1116:bool)  [unwired: 1 in, 5 out]
        n578 = case shown="True" w1116 {
          frame False {
          }
          frame True {
            n579 = local read "Measurement File"() -> (w1117:path)
            n580 = Two Button Dialog(message="Do you want to create additional files for the sweeping measurements?" ("string"), 1:"No" ("F button name (\"Cancel\")"), 2:"Yes" ("T button name (\"OK\")")) -> (T button?=w1119:bool)
            n581 = case shown="True" w1119 {
              tunnel: w1117 -> [_ w1124]
              frame False {
                n582 = local write "SaveSweep"(FALSE ("SaveSweep")) -> ()
              }
              frame True {
                n583 = call "Create_sweep_files.vi"("Measurement File"=w1124) -> ("Path 3"=→"Measurement File_dn":path, "Path 2"=→"Measurement File_up":path, "Path"=→"Measurement File_average":path)  [unwired: 8 in]
                "SaveSweep" <- TRUE
              }
            }
          }
        }
      }
      event "Measure Noise": Value Change {
        n584 = event-data() -> ("NewVal"=w1131:bool)  [unwired: 1 in, 5 out]
        n585 = case shown="True" w1131 {
          frame False {
          }
          frame True {
            n586 = local read "Gain (V/A)"() -> (w1136:dbl)
            n587 = call "Noise_measurement.vi"("Gain (V/A)"=w1136, "Cycles"="Cycles", "Lower Cut-Off"="Cut-Off Frequency", "minimum value"="minimum value", "Filter On"="Filter On", "maximum value"="maximum value", "physical channels"="physical channels", "rate"="Rate", "samples per channel"="Samples per channel") -> ("Current (pA) Filtered"=→"Current (pA) Filtered":waveform(dbl), "PSD (pA/Hz^1/2) Peaks Removed"=→"PSD (pA/Hz^1/2) Peaks Removed":cluster{"f0":dbl, "df":dbl, "magnitude":dbl[]}, "Current (pA)"=→"Current (pA)":dbl[], "PSD (pA/Hz^1/2)"=→"PSD (pA/Hz^1/2)":cluster{"f0":dbl, "df":dbl, "magnitude":dbl[]})  [unwired: 3 in]
          }
        }
      }
      event "Calibrate": Value Change {
        n588 = event-data() -> ()  [unwired: 1 in, 6 out]
        n589 = case shown="True" "Calibrate" {
          frame False {
          }
          frame True {
            w1149 = dbl[] []
            n590 = while {
              shift-right: [w1165] -> _
              shift-left: w1149 -> [w1166]
              shift-right: [w1159] -> _
              shift-left: w1149 -> [w1160]
              shift-right: [w1162] -> _
              shift-left: _ -> [w1161]
              tunnel: [w1157] -> w1150
              stop <- w1167 stop-if-true
              n591 = call "Calibration_Hall.vi"("Dwell Time (ms)"="Dwell Time (ms)", "R array in (V)"=w1160, "B array in (T)"=w1166, "Set Field (T)"=w1161, "dB"="dB") -> ("R array out (V)"=w1159:dbl[], "Ready?"=w1169:bool, 14:"Calibration Curve"=w1157:dbl[][], 15:"Calibration Curve"=→"Calibration Curve":cluster{dbl[], dbl[]}[], "B array Out"=w1165:dbl[], "Set Field out"=w1162:dbl)  [unwired: 9 in]
              "Calibration Curve Data" <- w1157
              n592 = Or(x=w1169, y="stop 2") -> (x .or. y?=w1167:bool)
            }
            n593 = flat-sequence {
              tunnel: w1150 -> [w1153]
              frame #0 {
                n594 = Two Button Dialog(message="Do you want to save calibration file?") -> (T button?=w1152:bool)  [unwired: 2 in]
                n595 = case shown="True" w1152 {
                  tunnel: w1153 -> [_ w1156]
                  frame False {
                  }
                  frame True {
                    n596 = Transpose 2D Array(2D array=w1156) -> (transposed array=w1154:dbl[][])
                    n597 = call-poly <vilib>:"Write Delimited Spreadsheet.vi"("format (%.3f)"="%.8f", "2D data"=w1154) -> ()  [unwired: 12 in, 2 out]
                  }
                }
              }
            }
          }
        }
      }
      event "New Measurement File": Value Change {
        n598 = event-data() -> ()  [unwired: 1 in, 6 out]
        n599 = local read "Sweep"() -> (w1171:bool)
        n600 = Open/Create/Replace File(prompt="Please select measurement file\n", operation (0:open)=T5."replace or create with confirmation") -> (refnum out=w1177:refnum<file>)  [unwired: 4 in, 2 out]
        n601 = local write "refnum out"(w1177) -> ()
        n602 = Refnum to Path(1:w1177) -> (0:w1172:path)
        n603 = case shown="True" w1171 {
          tunnel: w1172 -> [_ w1180]
          frame False {
          }
          frame True {
            n604 = Two Button Dialog(message="Do you want to create additional files for the sweeping measurements?" ("string"), 1:"No" ("F button name (\"Cancel\")"), 2:"Yes" ("T button name (\"OK\")")) -> (T button?=w1182:bool)
            n605 = case shown="True" w1182 {
              tunnel: w1180 -> [_ w1190]
              frame False {
                n606 = local write "SaveSweep"(FALSE ("SaveSweep")) -> ()
              }
              frame True {
                n607 = call "Create_sweep_files.vi"("Measurement File"=w1190) -> ("Path 3"=w1187:path, "Path 2"=w1188:path, "Path"=w1189:path)  [unwired: 8 in]
                n608 = local write "Measurement File_dn"(w1187) -> ()
                n609 = local write "Measurement File_average"(w1189) -> ()
                n610 = local write "Measurement File_up"(w1188) -> ()
                n611 = local write "SaveSweep"(TRUE) -> ()
              }
            }
          }
        }
        n612 = local write "Measurement File"(w1172) -> ()
        n613 = local write "Offset?"(FALSE ("Offset?")) -> ()
        n614 = local write "First?"(TRUE ("First?")) -> ()
      }
      event "Heater On/Off": Value Change {
        n615 = event-data() -> ()  [unwired: 1 in, 6 out]
        n616 = case shown="False" "Heater On/Off" {
          tunnel: w1195 -> [w1200 w1206]
          tunnel: w1194 -> [w1198 w1207]
          tunnel: [w1197 w1205] -> w1193
          frame False {
            n617 = VISA Write(VISA resource name=w1200, write buffer="RANGE,1,0", error in (no error)=w1198) -> (error out=w1197:errorcluster)  [unwired: 2 out]
          }
          frame True {
            n618 = Number To Decimal String(number="Heater Range") -> (decimal integer string=w1203:string)  [unwired: 1 in]
            n619 = Concatenate Strings("RANGE,1," ("write buffer"), w1203) -> (w1201:string)
            n620 = VISA Write(VISA resource name=w1206, write buffer=w1201, error in (no error)=w1207) -> (error out=w1205:errorcluster)  [unwired: 2 out]
          }
        }
      }
      event "Set temperature (K)": Value Change {
        n621 = event-data() -> ()  [unwired: 1 in, 6 out]
        n622 = local read "Set temperature (K)"() -> (w1213:dbl)
        n623 = Number To Fractional String(number=w1213, precision (6)=i16 3) -> (F-format string=w1216:string)  [unwired: 2 in]
        n624 = Concatenate Strings("SETP 1," ("write buffer"), w1216) -> (w1214:string)
        n625 = VISA Write(VISA resource name=w1210, write buffer=w1214, error in (no error)=w1212) -> (error out=w1211:errorcluster)  [unwired: 2 out]
      }
      event "Temp Ramping Rate (K/min)": Value Change {
        n626 = event-data() -> ()  [unwired: 1 in, 6 out]
        n627 = local read "Temp Ramping Rate (K/min)"() -> (w1220:dbl)
        n628 = Number To Fractional String(number=w1220, precision (6)=i16 1) -> (F-format string=w1226:string)  [unwired: 2 in]
        n629 = Concatenate Strings("RAMP 1,1," ("string"), w1226) -> (w1225:string)
        n630 = VISA Write(VISA resource name=w1223, write buffer=w1225, error in (no error)=w1222) -> (error out=w1221:errorcluster)  [unwired: 2 out]
      }
      event "Heater Range": Value Change {
        n631 = event-data() -> ()  [unwired: 1 in, 6 out]
        n632 = local read "Heater On/Off"() -> (w1232:bool)
        n633 = case shown="True" w1232 {
          tunnel: w1231 -> [w1233 w1238]
          tunnel: [w1233 w1237] -> w1230
          tunnel: w1228 -> [_ w1236]
          frame False {
          }
          frame True {
            n634 = local read "Heater Range"() -> (w1234:enum16{"Off", "Low", "Medium", "High"})
            n635 = Number To Decimal String(number=w1234) -> (decimal integer string=w1240:string)  [unwired: 1 in]
            n636 = Concatenate Strings("RANGE,1," ("write buffer"), w1240) -> (w1239:string)
            n637 = VISA Write(VISA resource name=w1236, write buffer=w1239, error in (no error)=w1238) -> (error out=w1237:errorcluster)  [unwired: 2 out]
          }
        }
      }
    }
    n638 = Reciprocal(x="Sampling rate (Hz)") -> (1/x=w907:dbl)
    n639 = Multiply(x=w907, y=1000.0) -> (x*y=w905:dbl)
    n640 = Wait Until Next ms Multiple(millisecond multiple=w905) -> ()  [unwired: 1 out]
  }
  n641 = local read "Max Field (T)"() -> (w72:dbl)
  n642 = local read "Min Field (T)"() -> (w74:dbl)
  n643 = local read "dB (T)"() -> (w73:dbl)
  n644 = Divide(x=w72, y=w73) -> (x/y=w75:dbl)
  n645 = for {
    N: w75 -> [_]
    tunnel: w73 -> [w1245]
    tunnel: [w1242] -> w35 mode=indexing
    tunnel: w74 -> [w1243]
    tunnel: [0.0] -> _ mode=indexing
    i -> [w1246]
    n646 = Multiply(x=w1246, y=w1245) -> (x*y=w1244:dbl)
    n647 = Add(x=w1244, y=w1243) -> (x+y=w1242:dbl)
  }
  n648 = Multiply(x=w35, y=0.0) -> (x*y=w32:dbl[])
  n649 = Array Size(array=w32) -> (size(s)=w31:i32)
  n650 = Decrement(x=w31) -> (x-1=w30:i32)
  n651 = local write "B array"(w35) -> ()
  n652 = Array Subset(array=w32, length=w30) -> (w29:dbl[])  [unwired: 1 in]
  n653 = Build Array(w32, w32) -> (w33:dbl[][])
  n654 = local read "Max temperature (K)"() -> (w1:dbl)
  n655 = local read "Min Temperature (K)"() -> (w3:dbl)
  n656 = local write "Averaged I(B)"(w33) -> ()
  n657 = Build Array(w29, w29) -> (w28:dbl[][])
  n658 = Divide(x=w1, y="dt (K)") -> (x/y=w5:dbl)
  n659 = local write "Averaged P(B)"(w28) -> ()
  n660 = local write "Averaged dt"(w28) -> ()
  n661 = for {
    N: w5 -> [_]
    tunnel: "dt (K)" -> [w1251]
    tunnel: [w1248] -> w4 mode=indexing
    tunnel: w3 -> [w1249]
    tunnel: [0.0] -> _ mode=indexing
    i -> [w1252]
    n662 = Multiply(x=w1252, y=w1251) -> (x*y=w1250:dbl)
    n663 = Add(x=w1250, y=w1249) -> (x+y=w1248:dbl)
  }
  "T array" <- w4
  n664 = local read "Lake Shore"() -> (w85:refnum<visa-resource-name>)
  n665 = local read "IV converter"() -> (w101:refnum<visa-resource-name>)
  n666 = local read "Magnetic Field"() -> (w100:refnum<visa-resource-name>)
  n667 = VISA Close(VISA resource name=w101, error in (no error)=w103) -> (error out=w104:errorcluster)
  n668 = VISA Close(VISA resource name=w100, error in (no error)=w104) -> (error out=w102:errorcluster)
  n669 = Release Queue(queue=w108, error in (no error)=w102) -> (error out=w98:errorcluster)  [unwired: 1 in, 2 out]
  n670 = Merge Errors(w98, w97) -> (w99:errorcluster)
  n671 = VISA Close(VISA resource name=w85, error in (no error)=w99) -> (error out=w96:errorcluster)
  n672 = local read "refnum out"() -> (w94:refnum<file>)
  n673 = Close File(refnum=w94, error in=w96) -> (error out=w95:errorcluster)  [unwired: 1 out]
  n674 = call <vilib>:"Simple Error Handler.vi"("error in (no error)"=w95) -> ()  [unwired: 4 in, 5 out]
  "i" <- w65
  "j" <- w65
